vi "ME_acquire_9.vi"() -> ()   [LabVIEW 2015]
doc: "Use this template to build a producer/consumer design pattern. Use this template when you need to execute a process, such as data analysis, when a data source, such as a triggered acquisition, produces data at an uneven rate and you need to execute the process when the data becomes available."
uses:
  Mode.ctl
  oxford_driver/Oxford Drivers/BUSGEN.LLB/OxfordAddress.ctl
  <vilib>/Analysis/baseanly.llb/Mean (DBL).vi
  <vilib>/Utility/file.llb/Write Delimited Spreadsheet (DBL).vi
  <vilib>/express/express arith-compare/Formula/XNode/ExpressFormulaBlockNode.xnode
  <vilib>/Analysis/NI_AALBase.lvlib
panel:
  out "remaining elements":T1(array[cluster])
  in  "Stop":bool
  out "SaveSweep":bool=TRUE
  out "Measurement File_dn":path
  out "Measurement File_up":path
  out "Measurement File_average":path
  out "Actual Polarization":dbl
  in  "Reset IB?":bool
  in  "First?":bool
  in  "Save Period":dbl=1.0
  out "Averaged I(B)":dbl[][](array[numeric])
  out "P(uC/mm^2)":dbl[](array[numeric])
  in  "Sweep Field":bool
  out "P(B)":cluster{"yi":dbl[], dbl[]}(graph)
  out "Offset array":dbl[](array[numeric])
  in  "stop 2":bool
  in  "dB":dbl=0.005
  in  "Dwell Time (ms)":u32=1
  out "appended array":dbl[][](array[numeric])
  in  "Magnet ON?":bool
  out "Actual B Field (T)":dbl
  out "Actual Temperature (K)":dbl
  out "Actual Current (pA)":dbl
  in  "Tab Control":T2(tab)
  out "P(T)":cluster{"yi":dbl[], dbl[]}(graph)
  out "I(T)":cluster{dbl[], dbl[]}(graph)
  in  "Set temperature (K)":dbl=4.5
  in  "Temp Ramping Rate (K/min)":dbl=10.0
  in  "Heater Range":enum16{"Off", "Low", "Medium", "High"}(ring)
  in  "Heater On/Off":bool
  in  "FileName":string
  out "Step Temp":bool
  out "j":i32
  out "i":i32
  in  "Max Countl":i32
  in  "Record ALL":bool
  in  "Sweep Rate Array":dbl[](array[numeric])=[2.0, 1.0, 0.5, 0.1, 0.05, 9.0, 10.0, 11.0, 12.0]
  out "I(B) 3":cluster{dbl[], dbl[]}[](graph)
  in  "Go to Set":bool
  in  "Set Field (T)":dbl
  in  "Field To Zero":bool
  in  "Sweep Rate (T/min)":dbl=2.0 format="%.6f"
  in  "Min Field (T)":dbl
  in  "Max Field (T)":dbl=0.15
  out "Up/Down":bool
  out "I(B) /Averaged/ 2":cluster{"B array":dbl[], dbl[]}[](graph)
  in  "Temperature Array":dbl[](array[numeric])=[4.5, 5.0, 6.0, 7.0, 8.0, 9.0, 10.0, 11.0, 12.0]
  out "New":bool=TRUE
  out "Step Rate":bool
  out "Finished":bool=TRUE
  in  "Directory":string
  out "Wait (s)":dbl
  in  "secs to wait":dbl=180.0
  in  "Measure Noise":bool
  in  "Cycles":i32
  in  "maximum value":dbl=10.0 format="%0.2f"
  in  "minimum value":dbl=-10.0 format="%0.2f"
  in  "physical channels":tag="Dev1/ai1"
  out "PSD (pA/Hz^1/2) Peaks Removed":cluster{"f0":dbl, "df":dbl, "magnitude":dbl[]}(graph)
  out "PSD (pA/Hz^1/2)":cluster{"f0":dbl, "df":dbl, "magnitude":dbl[]}(graph)
  out "Current (pA) Filtered":waveform(dbl)(graph)
  out "Current (pA)":dbl[](graph)
  in  "Samples per channel":i32=1000
  in  "Rate":dbl=1000.0 format="%0.2f"
  in  "Cut-Off Frequency":dbl=100.0 caption="Lower Cut-Off"
  in  "Filter On":bool
  out "Dc offset":dbl
  in  "Calibrate":bool
  in  "IV converter":refnum<visa-resource-name>="GPIB0::20::INSTR"
  in  "Magnetic Field":refnum<visa-resource-name>="GPIB0::21::INSTR"
  out "Time Lag":dbl=0.0500025749206543
  in  "Lake Shore":refnum<visa-resource-name>="GPIB0::11::INSTR"
  in  "Temp Refresh (s)":dbl=0.1
  in  "Sampling rate (Hz)":dbl=10.0
  in  "Gain (V/A)":dbl=1000000000.0
  in  "Sample area (mm^2)":dbl=3.9
  out "B_V":cluster{dbl[], "Best Linear Fit":dbl[]}[](graph)=[{[-0.00854253601, 0.00626134724, 0.0219834428, 0.0379117736, 0.0535871506, 0.0694316728, 0.0851615152, 0.100816481, 0.116478038, 0.132148461, 0.147876163, 0.16341701, 0.178976744, 0.194563632, 0.210251739, 0.225738944, 0.241298253, 0.256806034, 0.272344374, 0.287933477, 0.303494709, 0.318997125, 0.334591297, 0.350146681, 0.365618053, 0.380940961, 0.39666457, 0.412213675, 0.427724671, 0.443221444, 0.458760641, 0.474360042, 0.489915118, 0.505330598, 0.520967119, 0.536347531, 0.551813711, 0.567441155, 0.582995861, 0.598507522, 0.614041988, 0.629563151, 0.645106262, 0.660611914, 0.676136149, 0.691553948, 0.7071244, 0.72262999, 0.738171137, 0.753700392, 0.76919513, 0.784778028, 0.800215944, 0.8156961, 0.831325434, 0.846852183, 0.862326812, 0.877819169, 0.893312568, 0.90888536, 0.924354789], "Best Linear Fit"=[0.0, 0.005, 0.01, 0.015, 0.02, 0.025, 0.03, 0.035, 0.04, 0.045, 0.05, 0.055, 0.06, 0.065, 0.07, 0.075, 0.08, 0.085, 0.09, 0.095, 0.1, 0.105, 0.11, 0.115, 0.12, 0.125, 0.13, 0.135, 0.14, 0.145, 0.15, 0.155, 0.16, 0.165, 0.17, 0.175, 0.18, 0.185, 0.19, 0.195, 0.2, 0.205, 0.21, 0.215, 0.22, 0.225, 0.23, 0.235, 0.24, 0.245, 0.25, 0.255, 0.26, 0.265, 0.27, 0.275, 0.28, 0.285, 0.29, 0.295, 0.3]}, {[-0.00854253601, 0.00626134724, 0.0219834428, 0.0379117736, 0.0535871506, 0.0694316728, 0.0851615152, 0.100816481, 0.116478038, 0.132148461, 0.147876163, 0.16341701, 0.178976744, 0.194563632, 0.210251739, 0.225738944, 0.241298253, 0.256806034, 0.272344374, 0.287933477, 0.303494709, 0.318997125, 0.334591297, 0.350146681, 0.365618053, 0.380940961, 0.39666457, 0.412213675, 0.427724671, 0.443221444, 0.458760641, 0.474360042, 0.489915118, 0.505330598, 0.520967119, 0.536347531, 0.551813711, 0.567441155, 0.582995861, 0.598507522, 0.614041988, 0.629563151, 0.645106262, 0.660611914, 0.676136149, 0.691553948, 0.7071244, 0.72262999, 0.738171137, 0.753700392, 0.76919513, 0.784778028, 0.800215944, 0.8156961, 0.831325434, 0.846852183, 0.862326812, 0.877819169, 0.893312568, 0.90888536, 0.924354789], "Best Linear Fit"=[-0.00022554388023060128, 0.004536267537808887, 0.009593430775915074, 0.014716931562355689, 0.01975906732634002, 0.024855610270593523, 0.029915265354287977, 0.03495083565949541, 0.03998852608757118, 0.045029068349812316, 0.05008803495326229, 0.055086897848955874, 0.060091835929837946, 0.06510550835596321, 0.07015173884687344, 0.07513334727738563, 0.08013814865293042, 0.08512637555172443, 0.0901244320467579, 0.09513881694893507, 0.10014423687592358, 0.10513073807087174, 0.11014675346564809, 0.1151502923271957, 0.12012680792099008, 0.1250555686413888, 0.1301132186920259, 0.13511473785283767, 0.14010399888730068, 0.14508868495702945, 0.1500870171143548, 0.15510471446726903, 0.16010815425765457, 0.16506669165212906, 0.17009632901003072, 0.1750435864450521, 0.18001843198211442, 0.1850451496356715, 0.19004847041199868, 0.1950379453501071, 0.20003475573578386, 0.20502728708357412, 0.21002687821664084, 0.21501442030211, 0.220007939788244, 0.2249672231113706, 0.22997560874002893, 0.23496313088260184, 0.23996209027618054, 0.24495722449359253, 0.24994125598600042, 0.2549536449902534, 0.25991939913989753, 0.2648987401917687, 0.26992606578200207, 0.2749203939204135, 0.2798979571595809, 0.2848812227804405, 0.2898648235706211, 0.2948739618827834, 0.2998498524919418]}]
  out "V_I":cluster{dbl[], "Best Linear Fit":dbl[]}[](graph)=[{[0.0, 0.035, 0.069, 0.104, 0.138, 0.173, 0.208, 0.242, 0.277, 0.311, 0.346, 0.38, 0.415, 0.45, 0.484, 0.519, 0.553, 0.588, 0.623, 0.657, 0.692, 0.726, 0.761, 0.796, 0.83, 0.865, 0.899, 0.934, 0.969, 1.003, 1.038, 1.072, 1.107, 1.141, 1.176, 1.211, 1.245, 1.28, 1.314, 1.349, 1.384, 1.418, 1.453, 1.487, 1.522, 1.557, 1.591, 1.626, 1.66, 1.695, 1.73, 1.764, 1.799, 1.833, 1.868, 1.902, 1.937, 1.972, 2.006, 2.041, 2.075], "Best Linear Fit"=[-0.00854253601, 0.00626134724, 0.0219834428, 0.0379117736, 0.0535871506, 0.0694316728, 0.0851615152, 0.100816481, 0.116478038, 0.132148461, 0.147876163, 0.16341701, 0.178976744, 0.194563632, 0.210251739, 0.225738944, 0.241298253, 0.256806034, 0.272344374, 0.287933477, 0.303494709, 0.318997125, 0.334591297, 0.350146681, 0.365618053, 0.380940961, 0.39666457, 0.412213675, 0.427724671, 0.443221444, 0.458760641, 0.474360042, 0.489915118, 0.505330598, 0.520967119, 0.536347531, 0.551813711, 0.567441155, 0.582995861, 0.598507522, 0.614041988, 0.629563151, 0.645106262, 0.660611914, 0.676136149, 0.691553948, 0.7071244, 0.72262999, 0.738171137, 0.753700392, 0.76919513, 0.784778028, 0.800215944, 0.8156961, 0.831325434, 0.846852183, 0.862326812, 0.877819169, 0.893312568, 0.90888536, 0.924354789]}, {[0.0, 0.035, 0.069, 0.104, 0.138, 0.173, 0.208, 0.242, 0.277, 0.311, 0.346, 0.38, 0.415, 0.45, 0.484, 0.519, 0.553, 0.588, 0.623, 0.657, 0.692, 0.726, 0.761, 0.796, 0.83, 0.865, 0.899, 0.934, 0.969, 1.003, 1.038, 1.072, 1.107, 1.141, 1.176, 1.211, 1.245, 1.28, 1.314, 1.349, 1.384, 1.418, 1.453, 1.487, 1.522, 1.557, 1.591, 1.626, 1.66, 1.695, 1.73, 1.764, 1.799, 1.833, 1.868, 1.902, 1.937, 1.972, 2.006, 2.041, 2.075], "Best Linear Fit"=[-0.007846580254753975, 0.007882153481927697, 0.02316149482613275, 0.03889022856281441, 0.054169569907019474, 0.06989830364370113, 0.08562703738038281, 0.10090637872458785, 0.11663511246126955, 0.1319144538054746, 0.14764318754215625, 0.1629225288863613, 0.17865126262304296, 0.19437999635972467, 0.2096593377039297, 0.22538807144061138, 0.24066741278481643, 0.25639614652149806, 0.27212488025817977, 0.2874042216023848, 0.3031329553390665, 0.31841229668327153, 0.3341410304199532, 0.3498697641566349, 0.3651491055008399, 0.3808778392375216, 0.39615718058172666, 0.4118859143184083, 0.42761464805509, 0.442893989399295, 0.45862272313597674, 0.4739020644801818, 0.48963079821686345, 0.5049101395610684, 0.5206388732977502, 0.5363676070344319, 0.5516469483786369, 0.5673756821153185, 0.5826550234595236, 0.5983837571962053, 0.6141124909328869, 0.629391832277092, 0.6451205660137737, 0.6603999073579787, 0.6761286410946604, 0.691857374831342, 0.7071367161755471, 0.7228654499122288, 0.7381447912564338, 0.7538735249931156, 0.7696022587297972, 0.7848816000740022, 0.8006103338106839, 0.815889675154889, 0.8316184088915707, 0.8468977502357756, 0.8626264839724573, 0.878355217709139, 0.893634559053344, 0.9093632927900257, 0.9246426341342309]}]
  out "B0 (T)":dbl=0.0025222449819540214
  out "B/V (T/V)":dbl=0.321659617116981
  out "I0 (A)":dbl=-0.007846580254753975
  out "V/I (Ohm)":dbl=0.44939239247661916
  in  "Offset?":bool
  in  "Temp/Magnetic Field":bool
  out "index":i8
  out "Read?":bool
  out "Magnetic Field (T)":dbl[](array[numeric])
  out "Reset":bool
  out "Measured Current (pA)":dbl[](array[numeric])
  out "Elapsed Time (s)":dbl[](array[numeric])
  out "Start time":timestamp
  in  "Enum":T3=enum."Process"
  out "B array":dbl[](array[numeric])
  in  "dB (T)":dbl=0.0025
  in  "Counter":i8
  out "L magnet (H)":dbl
  out "R magnet (mOhm)":dbl
  out "Actual Current (R0)":dbl
  out "Actual Field (T)":dbl
  out "Temperature array":dbl[](array[numeric])
  in  "New Measurement File":bool
  out "Measurement File":path
  out "refnum out":refnum<file>
  in  "Measuring":bool
  in  "Measure /Pause":bool
  in  "stop":bool
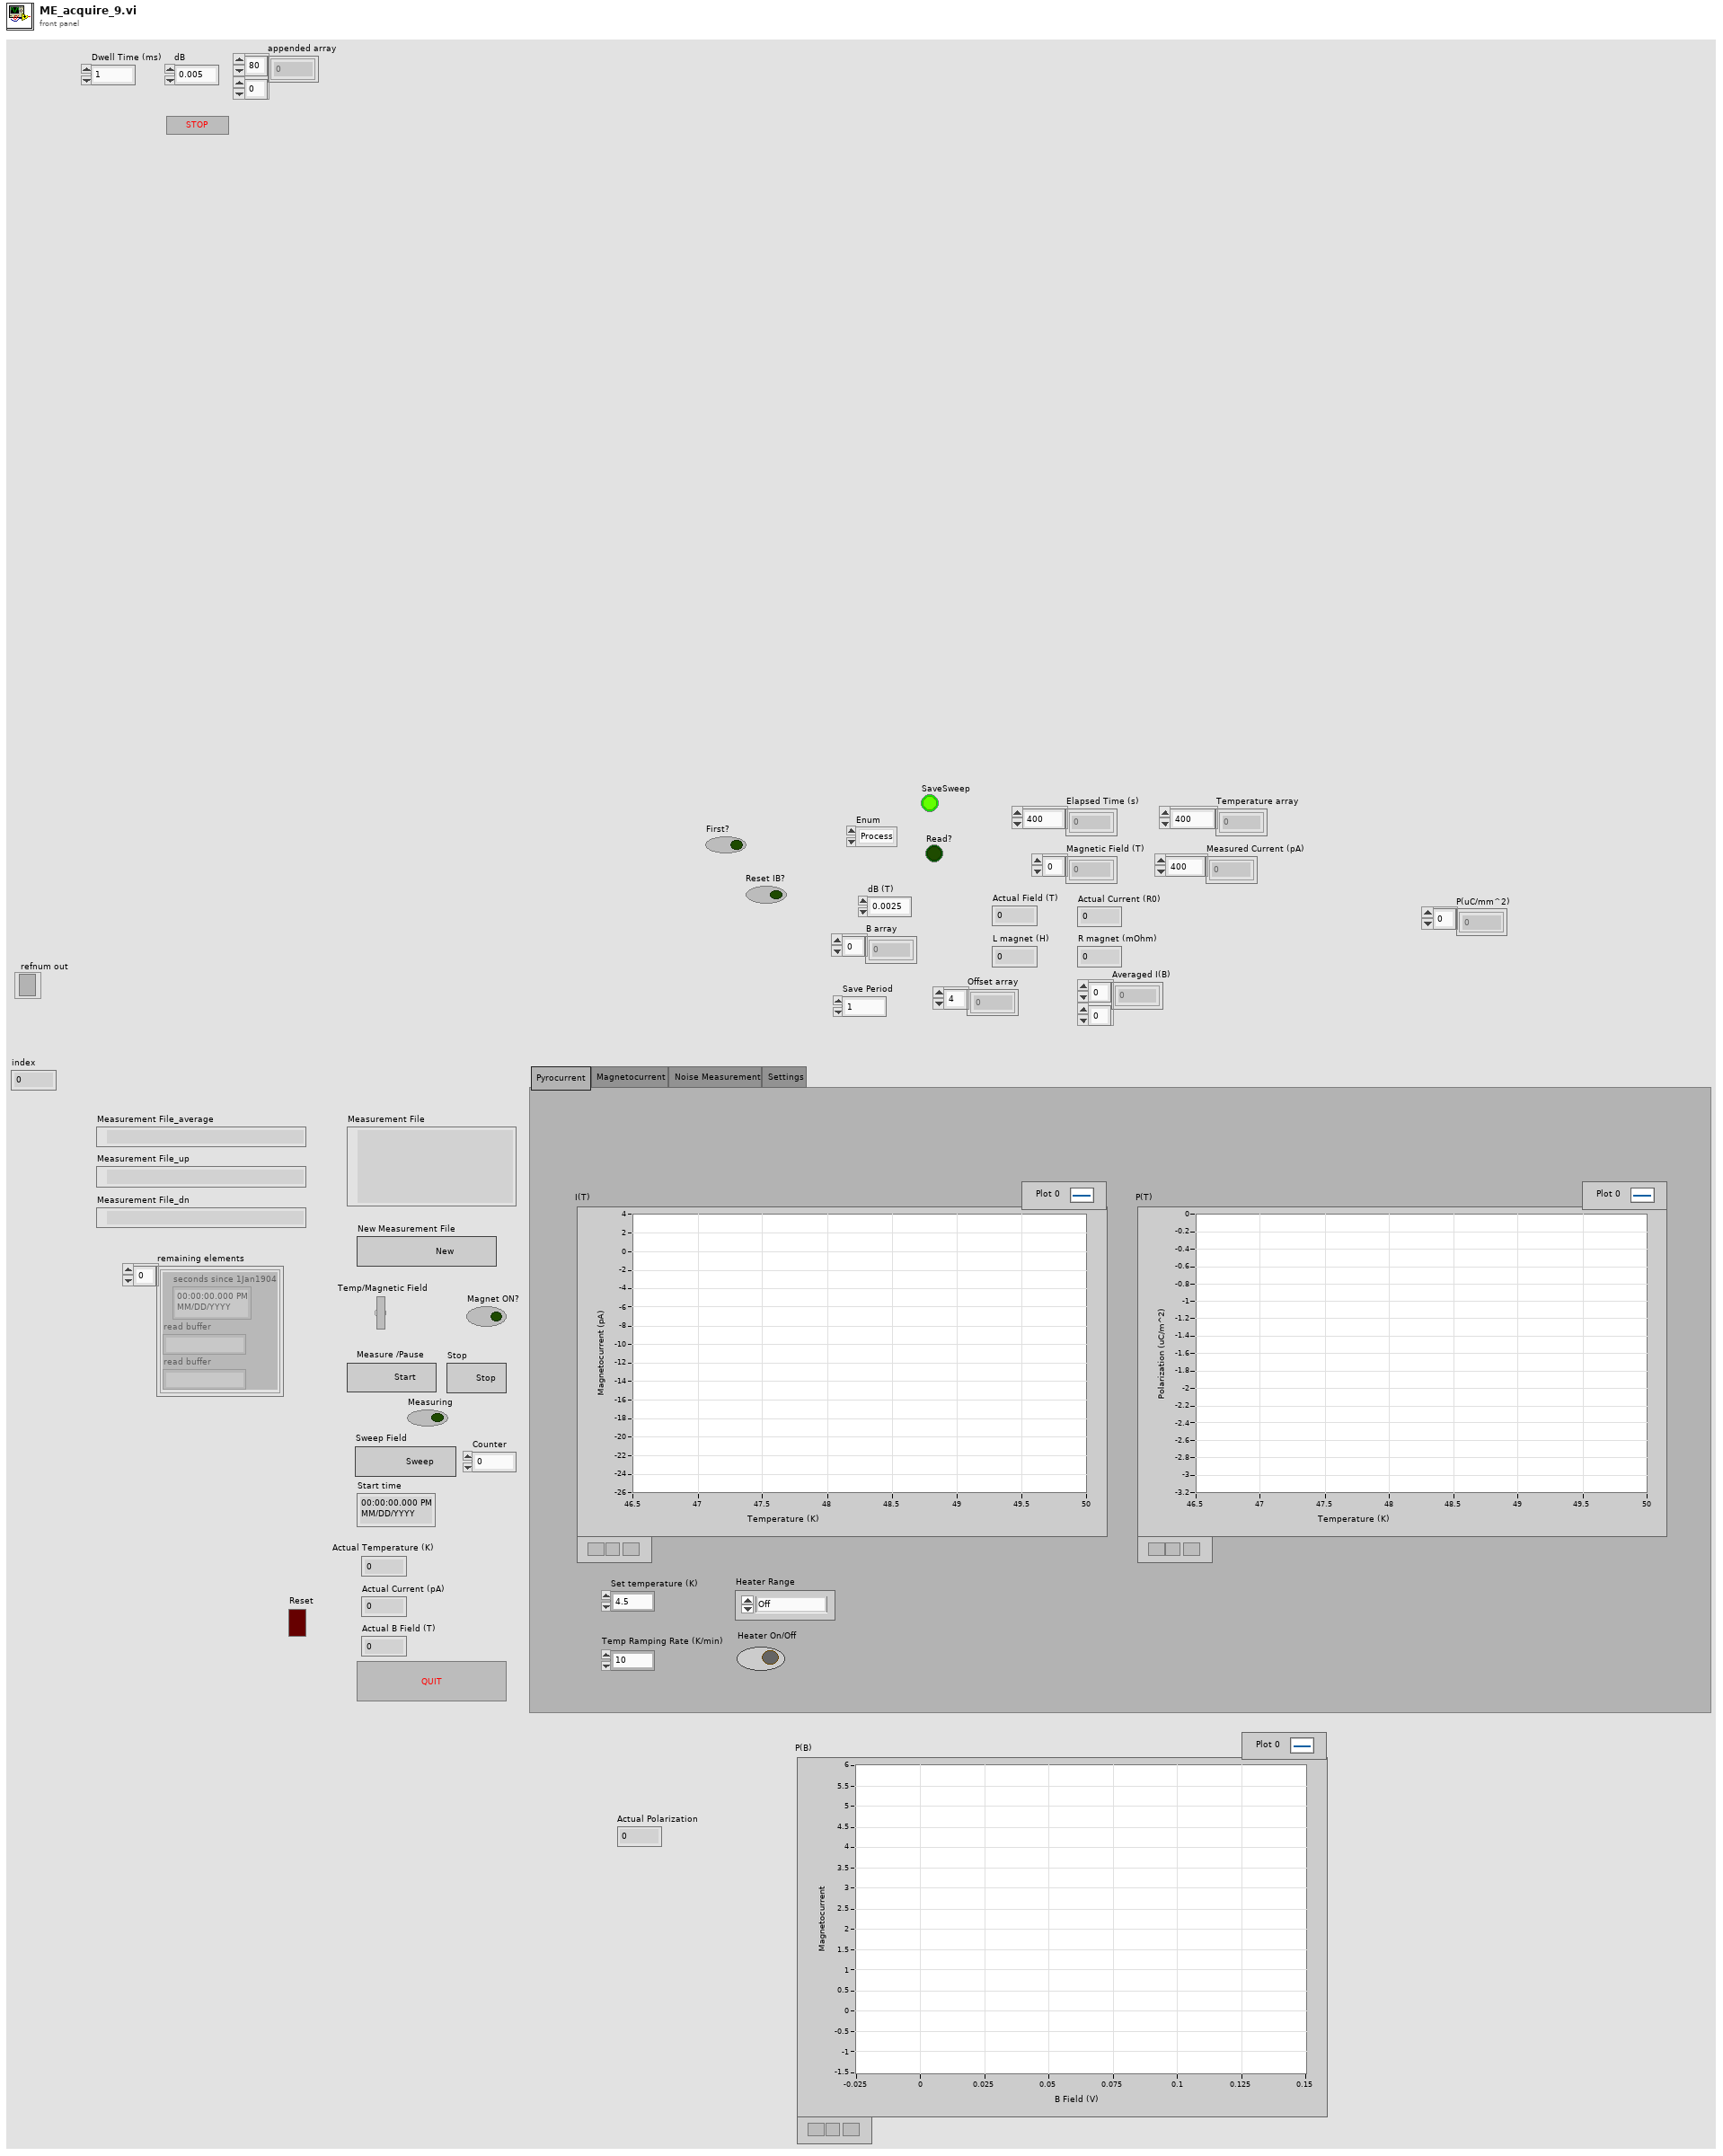
[diagram p1: front panel]
types:
  T1 = cluster{"seconds since 1Jan1904":timestamp, "read buffer":string, "read buffer":string}[]
  T2 = enum32{"Pyrocurrent", "Magnetocurrent", "Noise Measurement", "Settings"}
  T3 = typedef "Mode.ctl" = enum16{"Offset", "Process", "Sweep", "Plot", "Save", "New", "Return", ""}
  T4 = enum16{"open", "replace", "create", "open or create", "replace or create", "replace or create with confirmation"}
  T5 = typedef "OxfordAddress.ctl" = cluster{"Com Port":i32, "ISOBUS Address":i32, "GPIB Address":i16, "Communication":enum16{"RS232", "ISOBUS", "GPIB", "Gateway"}}
  T6 = cluster{"seconds since 1Jan1904":timestamp, "read buffer":string, "read buffer":string}
  T7 = cluster{"B array":dbl[], "Averaged I(B) out":dbl[]}
  T8 = cluster{"B array":dbl[], "Averaged I(B) out":dbl[]}[]
  T9 = cluster{"I array out (A)":dbl[], "V array out (V)":dbl[]}
  T10 = cluster{"I array out (A)":dbl[], "Best Linear Fit":dbl[]}
  T11 = cluster{"V array out (V)":dbl[], "B array Out":dbl[]}
  T12 = cluster{"V array out (V)":dbl[], "Best Linear Fit 2":dbl[]}
  T13 = cluster{"I array out (A)":dbl[], "Best Linear Fit":dbl[]}[]
  T14 = cluster{"V array out (V)":dbl[], "Best Linear Fit 2":dbl[]}[]
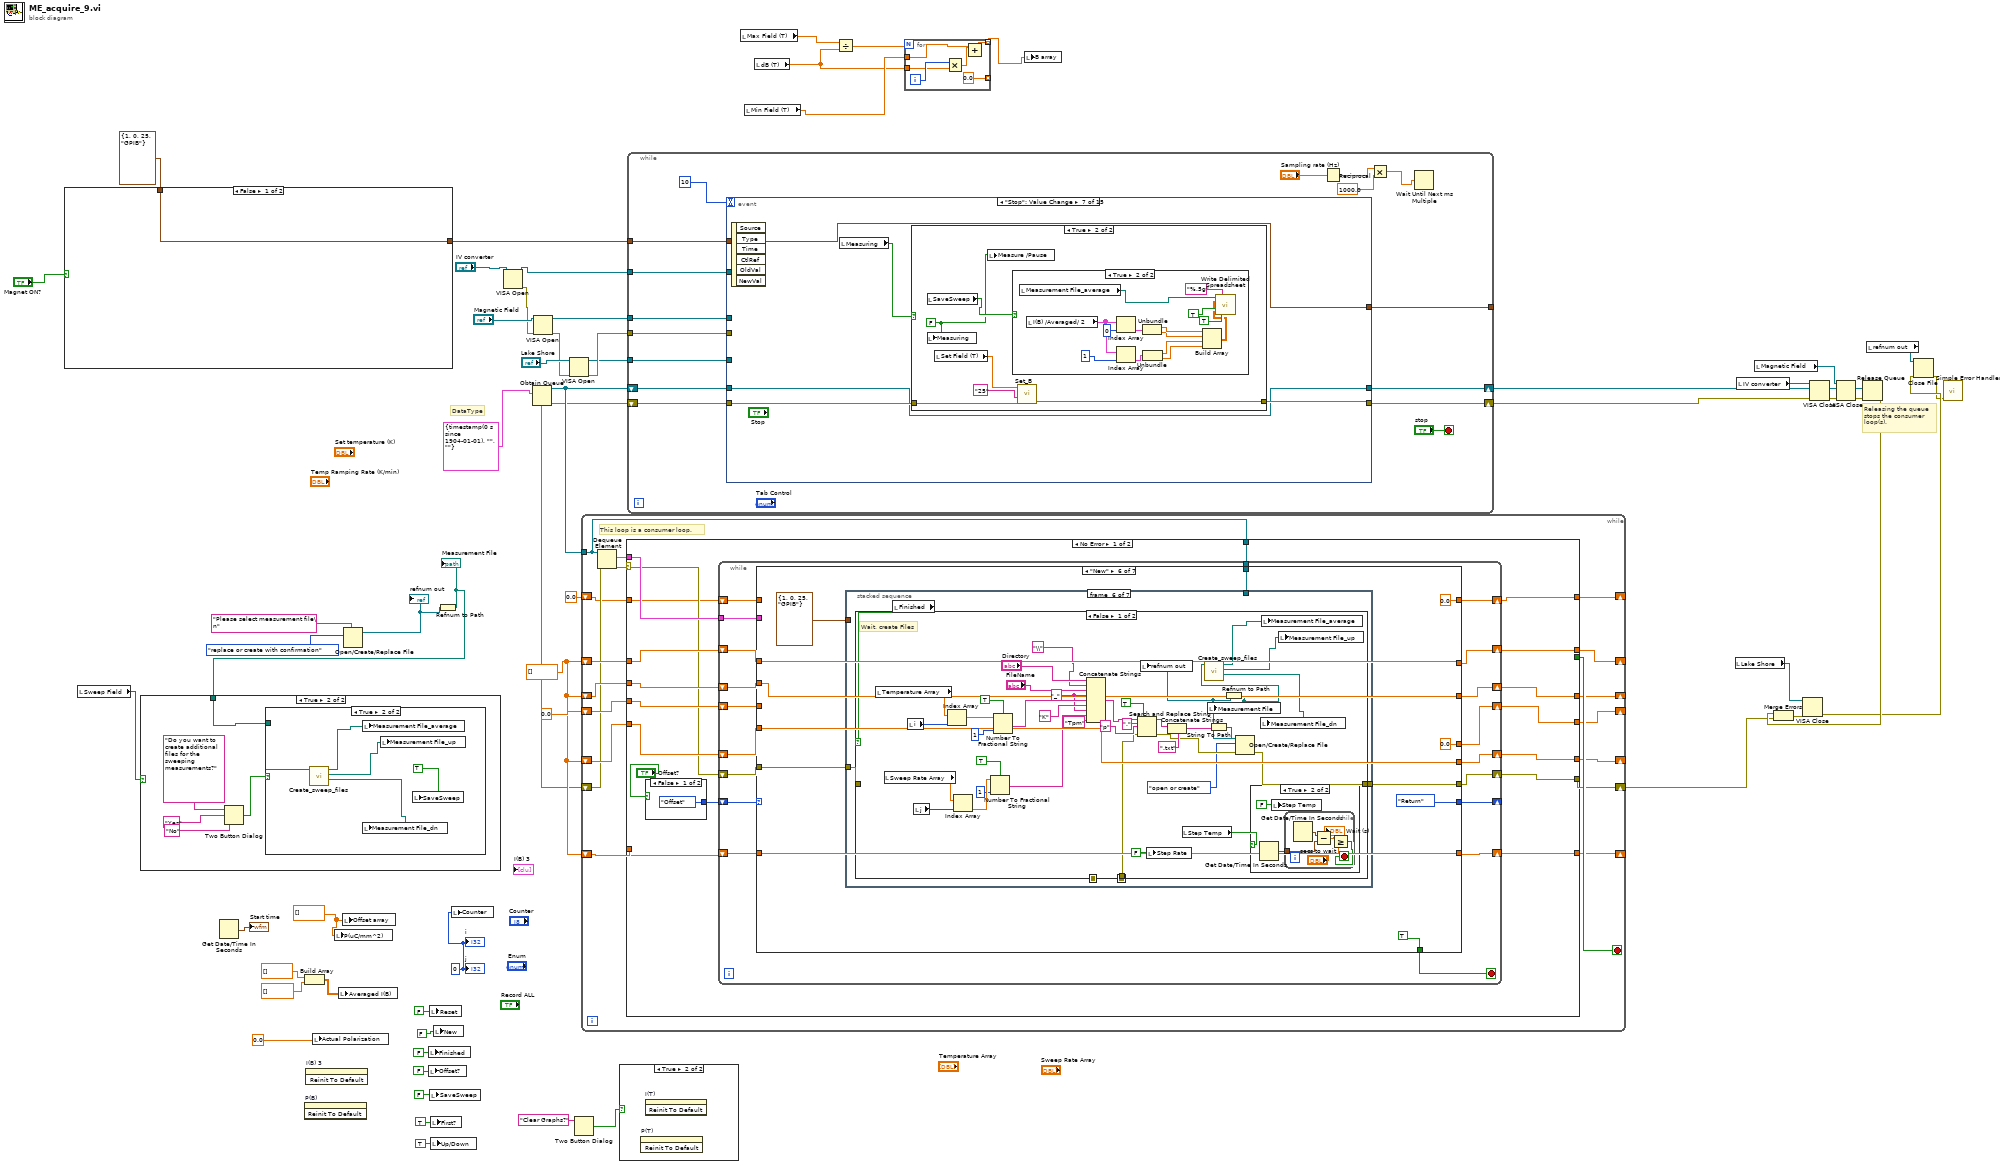
[diagram p0: block diagram]
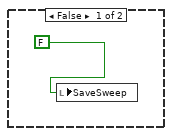
[diagram p4: hidden frame]
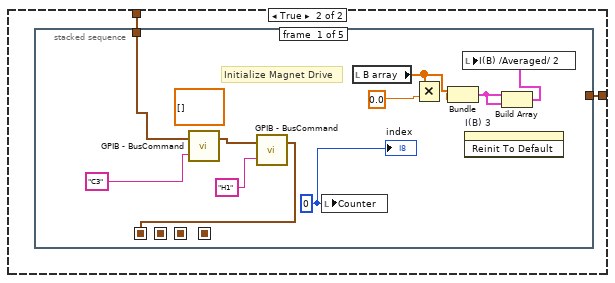
[diagram p5: hidden frame]
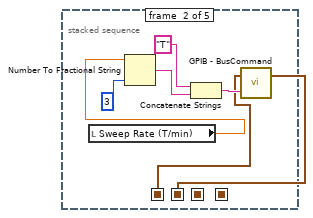
[diagram p6: hidden frame]
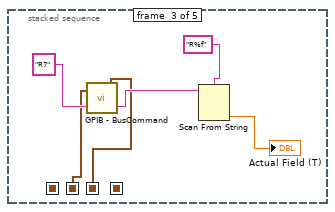
[diagram p7: hidden frame]
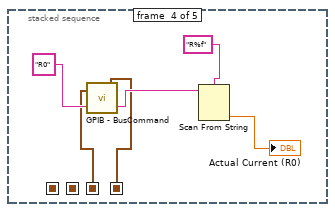
[diagram p8: hidden frame]
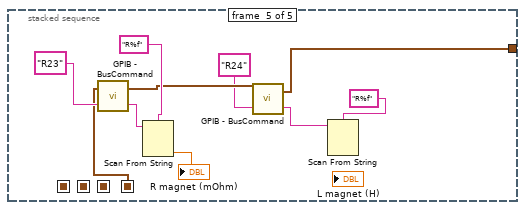
[diagram p9: hidden frame]
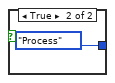
[diagram p10: hidden frame]
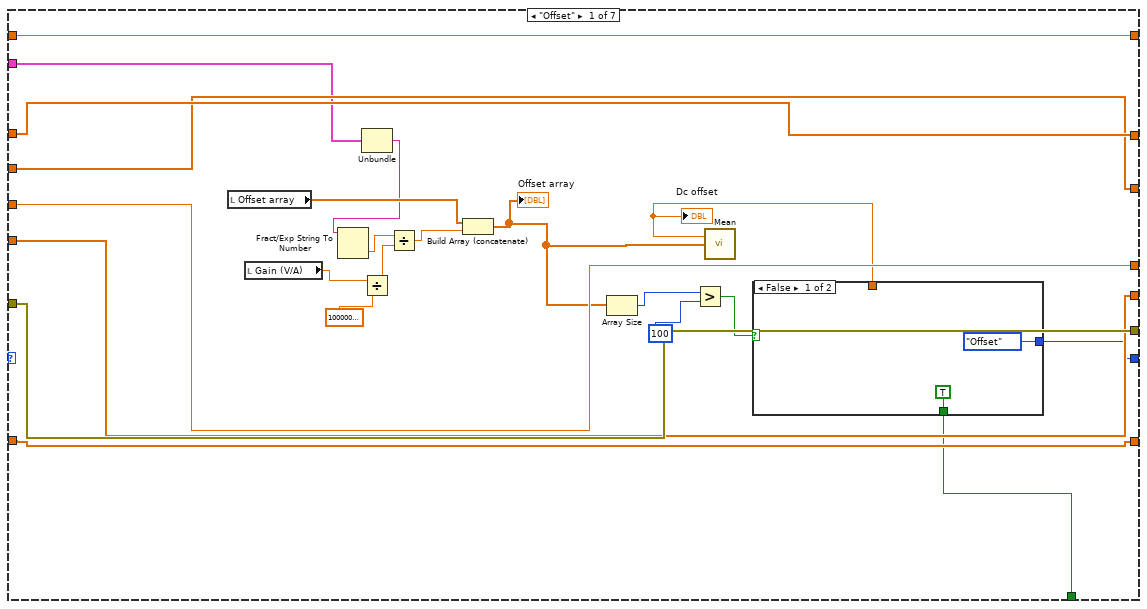
[diagram p11: hidden frame]
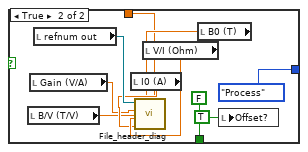
[diagram p12: hidden frame]
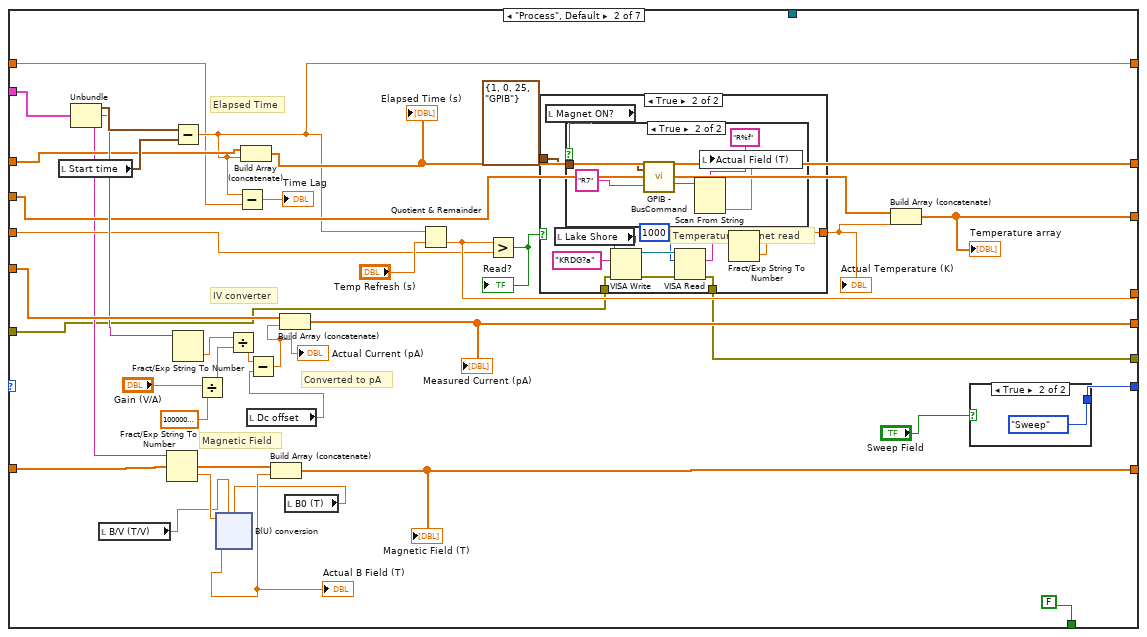
[diagram p13: hidden frame]
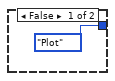
[diagram p14: hidden frame]
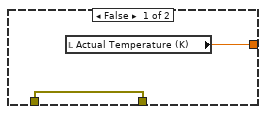
[diagram p15: hidden frame]
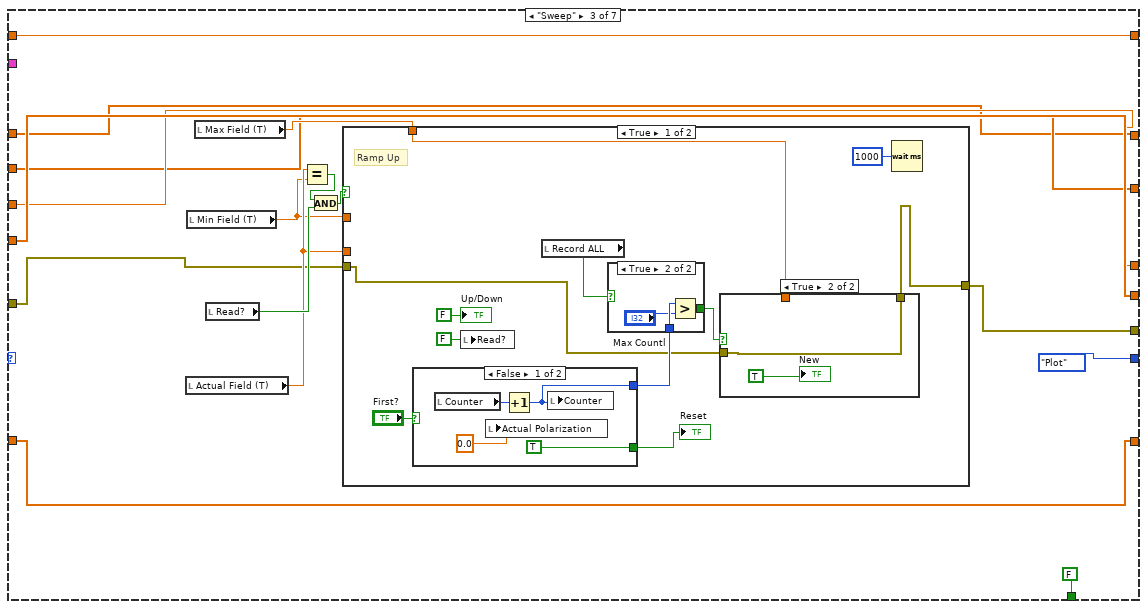
[diagram p17: hidden frame]
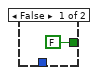
[diagram p18: hidden frame]
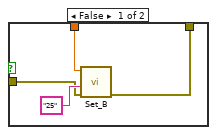
[diagram p19: hidden frame]
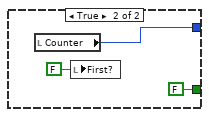
[diagram p20: hidden frame]
diagram:
  w3 = 0 ("j")
  w22 = dbl[] []
  w28 = dbl[] []
  # "DataType"
  # "Releasing the queue stops the consumer loop(s)."
  n1 = case shown="False" "Magnet ON?" {
    tunnel: T5 {"Com Port"=1, "ISOBUS Address"=0, "GPIB Address"=25, "Communication"=enum."GPIB"} ("Address") -> [w58 w60]
    tunnel: [w58 w59] -> w36
    frame False {
    }
    frame True {
      n2 = stacked-sequence {
        seq-local: [w68 _ _ _ _] -> [_ w73 _ _ _]
        seq-local: [_ w72 _ _ _] -> [_ _ w80 _ _]
        seq-local: [_ _ w79 _ _] -> [_ _ _ w86 _]
        seq-local: [_ _ _ w85 _] -> [_ _ _ _ w96]
        tunnel: w60 -> [w70 _ _ _ _]
        tunnel: [_ _ _ _ w94] -> w59
        frame #0 {
          (unwired) dbl[][] []
          w66 = i8 0 ("Counter")
          # "Initialize Magnet Drive"
          n3 = call "GPIB - BusCommand.vi"("Command"="C3", "Address"=w70) -> ("Address(thru)"=w69:T5)  [unwired: 1 out]
          n4 = call "GPIB - BusCommand.vi"("Command"="H1", "Address"=w69) -> ("Address(thru)"=w68:T5)  [unwired: 1 out]
          n5 = local write "Counter"(w66) -> ()
          n6 = local read "B array"() -> (w64:dbl[])
          n7 = Multiply(x=w64, y=0.0) -> (x*y=w63:dbl[])
          n8 = Bundle("B array"=w64, w63) -> (w62:cluster{"B array":dbl[], dbl[]})  [unwired: 1 in]
          n9 = invoke on="I(B) 3" class="XYGraph (strict)" method="Reinit To Default"() -> ()  [unwired: 3 in, 3 out]
          n10 = Build Array(w62, w62) -> (w61:cluster{"B array":dbl[], dbl[]}[])
          n11 = local write "I(B) /Averaged/ 2"(w61) -> ()
          "index" <- w66
        }
        frame #1 {
          n12 = local read "Sweep Rate (T/min)"() -> (w74:dbl)
          n13 = Number To Fractional String(number=w74, precision (6)=i16 3) -> (F-format string=w76:string)  [unwired: 2 in]
          n14 = Concatenate Strings("T" ("format string"), w76) -> (w75:string)
          n15 = call "GPIB - BusCommand.vi"("Command"=w75, "Address"=w73) -> ("Address(thru)"=w72:T5)  [unwired: 1 out]
        }
        frame #2 {
          n16 = call "GPIB - BusCommand.vi"("Command"="R7" ("format string"), "Address"=w80) -> ("Reply"=w84:string, "Address(thru)"=w79:T5)
          n17 = Scan From String(format string="R%f" ("remaining string"), input string=w84) -> (output 1=→"Actual Field (T)":dbl)  [unwired: 3 in, 3 out]
        }
        frame #3 {
          n18 = call "GPIB - BusCommand.vi"("Command"="R0" ("format string"), "Address"=w86) -> ("Reply"=w90:string, "Address(thru)"=w85:T5)
          n19 = Scan From String(format string="R%f" ("remaining string"), input string=w90) -> (output 1=→"Actual Current (R0)":dbl)  [unwired: 3 in, 3 out]
        }
        frame #4 {
          n20 = call "GPIB - BusCommand.vi"("Command"="R23" ("format string"), "Address"=w96) -> ("Reply"=w100:string, "Address(thru)"=w95:T5)
          n21 = Scan From String(format string="R%f" ("remaining string"), input string=w100) -> (output 1=→"R magnet (mOhm)":dbl)  [unwired: 3 in, 3 out]
          n22 = call "GPIB - BusCommand.vi"("Command"="R24" ("format string"), "Address"=w95) -> ("Reply"=w92:string, "Address(thru)"=w94:T5)
          n23 = Scan From String(format string="R%f" ("remaining string"), input string=w92) -> ()  [unwired: 4 in, 3 out]
        }
      }
    }
  }
  n24 = local read "Sweep Field"() -> (w8:bool)
  n25 = Get Date/Time In Seconds() -> (seconds since 1Jan1904=→"Start time":timestamp)
  n26 = Build Array(dbl[] [], dbl[] []) -> (w19:dbl[][])
  n27 = invoke on="P(B)" class="XYGraph (strict)" method="Reinit To Default"() -> ()  [unwired: 3 in, 3 out]
  n28 = invoke on="I(B) 3" class="XYGraph (strict)" method="Reinit To Default"() -> ()  [unwired: 3 in, 3 out]
  n29 = local write "Actual Polarization"(0.0 ("Actual Polarization")) -> ()
  n30 = local write "P(uC/mm^2)"(w22) -> ()
  n31 = local write "Averaged I(B)"(w19) -> ()
  n32 = local write "Offset array"(w22) -> ()
  n33 = Open/Create/Replace File(prompt="Please select measurement file\n", operation (0:open)=T4."replace or create with confirmation") -> (refnum out=w33:refnum<file>)  [unwired: 4 in, 2 out]
  "refnum out" <- w33
  n34 = local write "Finished"(FALSE ("Finished")) -> ()
  n35 = local write "Offset?"(FALSE ("Offset?")) -> ()
  n36 = local write "Reset"(FALSE ("Reset")) -> ()
  n37 = local write "SaveSweep"(FALSE ("SaveSweep")) -> ()
  n38 = local write "First?"(TRUE ("First?")) -> ()
  n39 = local write "Up/Down"(TRUE ("Up/Down")) -> ()
  n40 = local write "New"(FALSE ("New")) -> ()
  n41 = Refnum to Path(1:w33) -> (0:w7:path)
  "Measurement File" <- w7
  n42 = case shown="True" w8 {
    tunnel: w7 -> [_ w101]
    frame False {
    }
    frame True {
      n43 = Two Button Dialog(message="Do you want to create additional files for the sweeping measurements?" ("string"), 1:"No" ("F button name (\"Cancel\")"), 2:"Yes" ("T button name (\"OK\")")) -> (T button?=w103:bool)
      n44 = case shown="True" w103 {
        tunnel: w101 -> [_ w111]
        frame False {
          n45 = local write "SaveSweep"(FALSE ("SaveSweep")) -> ()
        }
        frame True {
          n46 = call "Create_sweep_files.vi"("Measurement File"=w111) -> ("Path 3"=w108:path, "Path 2"=w109:path, "Path"=w110:path)  [unwired: 8 in]
          n47 = local write "Measurement File_dn"(w108) -> ()
          n48 = local write "Measurement File_average"(w110) -> ()
          n49 = local write "Measurement File_up"(w109) -> ()
          n50 = local write "SaveSweep"(TRUE) -> ()
        }
      }
    }
  }
  n51 = local write "Counter"(w3) -> ()
  n52 = VISA Open(VISA resource name="IV converter") -> (VISA resource name=w52:refnum<visa-resource-name>, error out=w54:errorcluster)  [unwired: 4 in]
  n53 = Obtain Queue(element data type=T6 {"seconds since 1Jan1904"=timestamp(0 s since 1904-01-01), "read buffer"="", "read buffer"=""} ("output cluster")) -> (queue out=w57:refnum<queue>, error out=w26:errorcluster)  [unwired: 4 in, 1 out]
  n54 = VISA Open(error in (no error)=w54, VISA resource name="Magnetic Field") -> (VISA resource name=w51:refnum<visa-resource-name>, error out=w30:errorcluster)  [unwired: 3 in]
  n55 = VISA Open(error in (no error)=w30, VISA resource name="Lake Shore") -> (VISA resource name=w24:refnum<visa-resource-name>, error out=w29:errorcluster)  [unwired: 3 in]
  n56 = Two Button Dialog(message="Clear Graphs?") -> (T button?=w2:bool)  [unwired: 2 in]
  n57 = while {
    tunnel: w57 -> [w112]
    shift-right: [w125] -> _
    shift-left: w28 -> [w124]
    shift-right: [w123] -> _
    shift-left: w28 -> [w122]
    shift-right: [w121] -> _
    shift-left: w28 -> [w120]
    shift-right: [w119] -> _
    shift-left: 0.0 -> [w118]
    shift-right: [w117] -> _
    shift-left: w28 -> [w116]
    shift-right: [w126] -> w41
    shift-left: w26 -> [w115]
    shift-right: [w114] -> _
    shift-left: 0.0 -> [w113]
    stop <- w127 stop-if-true
    # "This loop is a consumer loop."
    n58 = Dequeue Element(queue=w112, error in (no error)=w115) -> (element=w128:T6, error out=w129:errorcluster)  [unwired: 1 in, 2 out]
    n59 = case shown="No Error" w129 {
      selector: w129 -> [w135 w640]
      tunnel: w128 -> [w146 _]
      tunnel: [_ TRUE] -> w127
      tunnel: [w134 w640] -> w126
      tunnel: [w145 w639] -> w125
      tunnel: w124 -> [w144 w639]
      tunnel: [w143 w636] -> w123
      tunnel: w122 -> [w142 w636]
      tunnel: [w141 w635] -> w121
      tunnel: w120 -> [w140 w635]
      tunnel: [w139 w637] -> w119
      tunnel: w118 -> [w138 w637]
      tunnel: [w137 w638] -> w117
      tunnel: w116 -> [w136 w638]
      tunnel: [w133 w634] -> w114
      tunnel: w113 -> [w132 w634]
      tunnel: w112 -> [w130 _]
      frame No Error {
        n60 = case shown="False" "Offset?" {
          tunnel: [Mode."Offset" ("Enum") Mode."Process" ("Enum")] -> w147
          frame False {
          }
          frame True {
          }
        }
        n61 = while {
          shift-right: [w156] -> _
          shift-left: w147 -> [w168]
          tunnel: w146 -> [w167]
          shift-right: [w166] -> w145
          shift-left: w144 -> [w165]
          shift-right: [w158] -> w137
          shift-left: w136 -> [w157]
          shift-right: [w160] -> w139
          shift-left: w138 -> [w159]
          shift-right: [w164] -> w143
          shift-left: w142 -> [w163]
          shift-right: [w154] -> w134
          shift-left: w135 -> [w155]
          shift-right: [w162] -> w141
          shift-left: w140 -> [w161]
          shift-right: [w152] -> w133
          shift-left: w132 -> [w151]
          tunnel: w130 -> [w150]
          stop <- w153 stop-if-true
          n62 = case shown="\"New\"" w168 {
            selector: w168 -> [_ _ _ _ _ _ w627]
            tunnel: w167 -> [w184 w238 _ _ _ _ _]
            tunnel: [w190 w235 w275 w343 w416 w484 w632] -> w166
            tunnel: w165 -> [w190 w226 w275 w343 w412 w484 w632]
            tunnel: [w185 w234 w278 w345 w418 w482 w629] -> w164
            tunnel: w163 -> [w185 w233 w278 w345 w413 w482 w629]
            tunnel: [w186 w230 w280 w340 w419 w480 w626] -> w162
            tunnel: w161 -> [w186 w229 w280 w340 w414 w480 w626]
            tunnel: [w188 w225 w277 w341 w422 0.0 w630] -> w160
            tunnel: w159 -> [w188 w224 w277 w341 w422 _ w630]
            tunnel: [w189 w221 w276 w342 w417 w483 w631] -> w158
            tunnel: w157 -> [w189 w222 w276 w342 w415 w483 w631]
            tunnel: [w173 w219 Mode."Plot" ("Enum") Mode."Save" ("Enum") w423 Mode."Return" ("Enum") w627] -> w156
            tunnel: w155 -> [w187 w217 w282 w348 w421 w476 w628]
            tunnel: [w187 w216 w281 w348 w421 w475 w628] -> w154
            tunnel: [w169 FALSE FALSE FALSE w410 TRUE TRUE] -> w153
            tunnel: [w172 w213 w274 w344 w420 0.0 w633] -> w152
            tunnel: w151 -> [w172 w212 w274 w344 w420 _ w633]
            tunnel: w150 -> [_ _ _ _ _ w474 _]
            frame "Offset" {
              n63 = local read "Offset array"() -> (w178:dbl[])
              n64 = local read "Gain (V/A)"() -> (w182:dbl)
              n65 = Unbundle(w184) -> ("read buffer"=w171:string)  [unwired: 2 out]
              n66 = Fract/Exp String To Number(string=w171) -> (number=w183:dbl)  [unwired: 3 in, 1 out]
              n67 = Divide(x=w182, y=1000000000000.0) -> (x/y=w180:dbl)
              n68 = Divide(x=w183, y=w180) -> (x/y=w179:dbl)
              n69 = Build Array (concatenate)(w178, w179) -> (w174:dbl[])
              "Offset array" <- w174
              n70 = Array Size(array=w174) -> (size(s)=w177:i32)
              n71 = Greater?(x=w177, y=100) -> (0:w175:bool)
              n72 = call-poly <vilib>:"Mean.vi"("X"=w174) -> ("mean"=w170:dbl)  [unwired: 1 out]
              "Dc offset" <- w170
              n73 = case shown="False" w175 {
                tunnel: [Mode."Offset" ("Enum") Mode."Process" ("Enum")] -> w173
                tunnel: w170 -> [_ w194]
                tunnel: [TRUE FALSE] -> w169
                frame False {
                }
                frame True {
                  n74 = local read "B/V (T/V)"() -> (w195:dbl)
                  n75 = local read "Gain (V/A)"() -> (w196:dbl)
                  n76 = local read "refnum out"() -> (w200:refnum<file>)
                  n77 = local read "I0 (A)"() -> (w198:dbl)
                  n78 = local read "V/I (Ohm)"() -> (w199:dbl)
                  n79 = local read "B0 (T)"() -> (w197:dbl)
                  n80 = call "File_header_diag.vi"("OFFSET"=w194, "B0"=w197, "B/V"=w195, "I0"=w198, "V/I"=w199, "Gain"=w196, "Byte Stream File in"=w200) -> ()  [unwired: 5 in]
                  n81 = local write "Offset?"(TRUE ("Offset?")) -> ()
                }
              }
            }
            frame "Process", Default {
              # "Converted to pA"
              # "Magnetic Field"
              # "IV converter"
              # "Elapsed Time"
              n82 = local read "Start time"() -> (w236:timestamp)
              n83 = Unbundle(w238) -> ("seconds since 1Jan1904"=w237:timestamp, "read buffer"=w231:string, "read buffer"=w218:string)
              n84 = local read "B/V (T/V)"() -> (w208:dbl)
              n85 = Fract/Exp String To Number(string=w218) -> (number=w228:dbl)  [unwired: 3 in, 1 out]
              n86 = Subtract(x=w237, y=w236) -> (x-y=w213:dbl)
              n87 = Fract/Exp String To Number(string=w231) -> (number=w232:dbl)  [unwired: 3 in, 1 out]
              n88 = Divide(x="Gain (V/A)", y=1000000000000.0) -> (x/y=w211:dbl)
              n89 = Divide(x=w232, y=w211) -> (x/y=w206:dbl)
              n90 = Subtract(x=w213, y=w212) -> (x-y=→"Time Lag":dbl)
              n91 = Build Array (concatenate)(w226, w213) -> (w235:dbl[])
              "Elapsed Time (s)" <- w235
              n92 = local read "Dc offset"() -> (w204:dbl)
              n93 = Subtract(x=w206, y=w204) -> (x-y=w205:dbl)
              "Actual Current (pA)" <- w205
              n94 = Build Array (concatenate)(w233, w205) -> (w234:dbl[])
              "Measured Current (pA)" <- w234
              n95 = local read "B0 (T)"() -> (w207:dbl)
              n96 = xnode "B(U) conversion"("V"=w228, "BpV"=w208, "B0"=w207) -> ("Result"=w227:dbl)  [unwired: 1 in, 1 out]
              "Actual B Field (T)" <- w227
              n97 = Build Array (concatenate)(w229, w227) -> (w230:dbl[])
              "Magnetic Field (T)" <- w230
              n98 = Quotient & Remainder(x=w213, y="Temp Refresh (s)") -> (floor(x/y)=w225:dbl)  [unwired: 1 out]
              n99 = Greater?(x=w225, y=w224) -> (0:w223:bool)
              "Read?" <- w223
              n100 = case shown="True" w223 {
                tunnel: [w244 w250] -> w220
                tunnel: w217 -> [w243 w249]
                tunnel: [w243 w248] -> w216
                tunnel: T5 {"Com Port"=1, "ISOBUS Address"=0, "GPIB Address"=25, "Communication"=enum."GPIB"} ("Address") -> [_ w247]
                frame False {
                  n101 = local read "Actual Temperature (K)"() -> (w244:dbl)
                }
                frame True {
                  # "Temperature/Magnet read"
                  n102 = local read "Magnet ON?"() -> (w245:bool)
                  n103 = local read "Lake Shore"() -> (w246:refnum<visa-resource-name>)
                  n104 = case shown="True" w245 {
                    tunnel: w247 -> [_ w257]
                    frame False {
                    }
                    frame True {
                      n105 = call "GPIB - BusCommand.vi"("Command"="R7" ("format string"), "Address"=w257) -> ("Reply"=w258:string)  [unwired: 1 out]
                      n106 = Scan From String(format string="R%f" ("remaining string"), input string=w258) -> (output 1=w256:dbl)  [unwired: 3 in, 3 out]
                      n107 = local write "Actual Field (T)"(w256) -> ()
                    }
                  }
                  n108 = VISA Write(VISA resource name=w246, write buffer="KRDG?a", error in (no error)=w249) -> (VISA resource name out=w254:refnum<visa-resource-name>, error out=w253:errorcluster)  [unwired: 1 out]
                  n109 = VISA Read(VISA resource name=w254, byte count=u32 1000, error in (no error)=w253) -> (read buffer=w251:string, error out=w248:errorcluster)  [unwired: 2 out]
                  n110 = Fract/Exp String To Number(string=w251) -> (number=w250:dbl)  [unwired: 3 in, 1 out]
                }
              }
              "Actual Temperature (K)" <- w220
              n111 = Build Array (concatenate)(w222, w220) -> (w221:dbl[])
              "Temperature array" <- w221
              n112 = case shown="True" "Sweep Field" {
                tunnel: [Mode."Plot" ("Enum") Mode."Sweep" ("Enum")] -> w219
                frame False {
                }
                frame True {
                }
              }
            }
            frame "Sweep" {
              n113 = local read "Actual Field (T)"() -> (w285:dbl)
              n114 = local read "Min Field (T)"() -> (w284:dbl)
              n115 = local read "Max Field (T)"() -> (w283:dbl)
              n116 = local read "Read?"() -> (w288:bool)
              n117 = Equal?(x=w285, y=w284) -> (x = y?=w286:bool)
              n118 = And(x=w286, y=w288) -> (x .and. y?=w287:bool)
              n119 = case shown="True" w287 {
                tunnel: [w292 w323] -> w281
                tunnel: w283 -> [w290 w322]
                tunnel: w284 -> [_ w321]
                tunnel: w285 -> [_ w319]
                tunnel: w282 -> [w293 w318]
                frame True {
                  # "Ramp Up"
                  n120 = case shown="False" "First?" {
                    tunnel: [TRUE ("Save") FALSE ("Save")] -> w296
                    tunnel: [w310 w314] -> w295
                    frame False {
                      n121 = local read "Counter"() -> (w313:i8)
                      n122 = local write "Actual Polarization"(0.0 ("Actual Polarization")) -> ()
                      n123 = Increment(x=w313) -> (x+1=w310:i8)
                      n124 = local write "Counter"(w310) -> ()
                    }
                    frame True {
                      n125 = local read "Counter"() -> (w314:i8)
                      n126 = local write "First?"(FALSE ("First?")) -> ()
                    }
                  }
                  "Reset" <- w296
                  n127 = local write "Read?"(FALSE ("Read?")) -> ()
                  n128 = local read "Record ALL"() -> (w291:bool)
                  n129 = case shown="True" w291 {
                    tunnel: w295 -> [_ w303]
                    tunnel: [FALSE w301] -> w294
                    frame False {
                    }
                    frame True {
                      n130 = Greater?(x=w303, y="Max Countl") -> (0:w301:bool)
                    }
                  }
                  n131 = case shown="True" w294 {
                    tunnel: w293 -> [w306 w309]
                    tunnel: [w305 w309] -> w292
                    tunnel: w290 -> [w304 _]
                    frame False {
                      n132 = call "Set_B.vi"("error in (no error)"=w306, "address string"="25", "Set Field (T)"=w304) -> ("error out"=w305:errorcluster)  [unwired: 8 in]
                    }
                    frame True {
                      "New" <- TRUE
                    }
                  }
                  n133 = Wait (ms)(milliseconds to wait=u32 1000) -> ()  [unwired: 1 out]
                  "Up/Down" <- FALSE ("Up/Down")
                }
                frame False {
                  n134 = Equal?(x=w322, y=w319) -> (x = y?=w320:bool)
                  n135 = case shown="True" w320 {
                    tunnel: [w324 w328] -> w323
                    tunnel: w321 -> [_ _]
                    tunnel: w318 -> [w324 w329]
                    frame False {
                    }
                    frame True {
                      # "Resetting at the end of every cycle"
                      # "Ramp Dn"
                      n136 = local write "Up/Down"(TRUE ("Up/Down")) -> ()
                      n137 = local read "Min Field (T)"() -> (w327:dbl)
                      n138 = call "Set_B.vi"("error in (no error)"=w329, "address string"="25", "Set Field (T)"=w327) -> ("error out"=w328:errorcluster)  [unwired: 8 in]
                      n139 = local write "Reset"(TRUE ("Reset")) -> ()
                      n140 = Wait (ms)(milliseconds to wait=u32 1000) -> ()  [unwired: 1 out]
                    }
                  }
                  n141 = local write "Read?"(FALSE ("Read?")) -> ()
                }
              }
            }
            frame "Plot" {
              # "dI"
              n142 = local read "P(uC/mm^2)"() -> (w333:dbl[])
              n143 = local read "Actual Polarization"() -> (w332:dbl)
              n144 = local read "Actual Current (pA)"() -> (w334:dbl)
              n145 = local read "Time Lag"() -> (w346:dbl)
              n146 = Multiply(x=w334, y=w346) -> (x*y=w338:dbl)
              n147 = Divide(x=w338, y="Sample area (mm^2)") -> (x/y=w337:dbl)
              n148 = Add(x=w337, y=w332) -> (x+y=w336:dbl)
              "Actual Polarization" <- w336
              n149 = local read "Temp/Magnetic Field"() -> (w347:bool)
              n150 = Build Array (concatenate)(w333, w336) -> (→"P(uC/mm^2)":dbl[])
              n151 = case shown="True" w347 {
                tunnel: w344 -> [_ w407]
                tunnel: w341 -> [_ w389]
                tunnel: w336 -> [w354 w390]
                frame False {
                  # "Magnetic Field plotting"
                  n152 = local read "Up/Down"() -> (w359:bool)
                  n153 = local read "Actual B Field (T)"() -> (w356:dbl)
                  n154 = case shown="False" w359 {
                    frame True {
                      # "Down"
                      n155 = local read "I(B) 3"() -> (w369:cluster{dbl[], dbl[]}[])
                      n156 = local read "I(B) 3"() -> (w373:cluster{dbl[], dbl[]}[])
                      n157 = Index Array(array=w369, index=1) -> (element=w367:cluster{dbl[], dbl[]})
                      n158 = Unbundle(w367) -> (w366:dbl[], w365:dbl[])
                      n159 = Index Array(array=w373, index=i8 0 ("t")) -> (element=w370:cluster{dbl[], dbl[]})
                      n160 = local read "Actual Current (pA)"() -> (w362:dbl)
                      n161 = local read "Actual B Field (T)"() -> (w361:dbl)
                      n162 = Build Array (concatenate)(w366, w361) -> (w364:dbl[])
                      n163 = Build Array (concatenate)(w365, w362) -> (w363:dbl[])
                      n164 = Bundle(w364, w363) -> (w360:cluster{dbl[], dbl[]})  [unwired: 1 in]
                      n165 = Build Array(w370, w360) -> (w371:cluster{dbl[], dbl[]}[])
                      n166 = local write "I(B) 3"(w371) -> ()
                    }
                    frame False {
                      # "Up"
                      n167 = local read "I(B) 3"() -> (w385:cluster{dbl[], dbl[]}[])
                      n168 = local read "I(B) 3"() -> (w387:cluster{dbl[], dbl[]}[])
                      n169 = Index Array(array=w385, index=0) -> (element=w383:cluster{dbl[], dbl[]})
                      n170 = Unbundle(w383) -> (w382:dbl[], w381:dbl[])
                      n171 = Index Array(array=w387, index=i8 1 ("t")) -> (element=w375:cluster{dbl[], dbl[]})
                      n172 = local read "Actual B Field (T)"() -> (w377:dbl)
                      n173 = local read "Actual Current (pA)"() -> (w376:dbl)
                      n174 = Build Array (concatenate)(w382, w377) -> (w380:dbl[])
                      n175 = Build Array (concatenate)(w381, w376) -> (w379:dbl[])
                      n176 = Bundle(w380, w379) -> (w378:cluster{dbl[], dbl[]})  [unwired: 1 in]
                      n177 = Build Array(w378, w375) -> (w374:cluster{dbl[], dbl[]}[])
                      n178 = local write "I(B) 3"(w374) -> ()
                    }
                  }
                  n179 = local read "P(B)"() -> (w358:cluster{"yi":dbl[], dbl[]})
                  n180 = Unbundle(w358) -> ("yi"=w357:dbl[], w355:dbl[])
                  n181 = Build Array (concatenate)(w357, w356) -> (w353:dbl[])
                  n182 = Build Array (concatenate)(w355, w354) -> (w352:dbl[])
                  n183 = Bundle(w353, w352) -> (→"P(B)":cluster{dbl[], dbl[]})  [unwired: 1 in]
                }
                frame True {
                  # "Temperature plotting"
                  n184 = Quotient & Remainder(x=w407, y="Save Period") -> (x-y*floor(x/y)=w388:dbl)  [unwired: 1 out]
                  n185 = Greater?(x=w389, y=w388) -> (0:w405:bool)
                  n186 = local read "Actual Temperature (K)"() -> (w392:dbl)
                  n187 = local read "Actual Current (pA)"() -> (w398:dbl)
                  n188 = local read "P(T)"() -> (w394:cluster{"yi":dbl[], dbl[]})
                  n189 = local read "I(T)"() -> (w404:cluster{dbl[], dbl[]})
                  n190 = case shown="True" w405 {
                    frame False {
                    }
                    frame True {
                      n191 = local write "Reset"(TRUE) -> ()
                    }
                  }
                  n192 = Unbundle(w394) -> ("yi"=w395:dbl[], w391:dbl[])
                  n193 = Unbundle(w404) -> (w402:dbl[], w401:dbl[])
                  n194 = Build Array (concatenate)(w395, w392) -> (w396:dbl[])
                  n195 = Build Array (concatenate)(w391, w390) -> (w397:dbl[])
                  n196 = Build Array (concatenate)(w402, w392) -> (w400:dbl[])
                  n197 = Build Array (concatenate)(w401, w398) -> (w399:dbl[])
                  n198 = Bundle(w400, w399) -> (→"I(T)":cluster{dbl[], dbl[]})  [unwired: 1 in]
                  n199 = Bundle(w396, w397) -> (→"P(T)":cluster{dbl[], dbl[]})  [unwired: 1 in]
                }
              }
            }
            frame "Save" {
              n200 = local read "Reset"() -> (w409:bool)
              n201 = case shown="True" w409 {
                tunnel: w414 -> [w431 w433]
                tunnel: [w431 w436] -> w419
                tunnel: w413 -> [w430 w434]
                tunnel: [w430 w436] -> w418
                tunnel: w415 -> [w429 w435]
                tunnel: [w429 w436] -> w417
                tunnel: [w428 w436] -> w416
                tunnel: w412 -> [w428 w432]
                frame False {
                }
                frame True {
                  n202 = stacked-sequence {
                    tunnel: [_ _ w473] -> w436
                    tunnel: w435 -> [_ w462 _]
                    tunnel: w434 -> [w447 w460 _]
                    tunnel: w433 -> [w448 w461 _]
                    tunnel: w432 -> [_ w458 _]
                    frame #0 {
                      n203 = local read "B array"() -> (w438:dbl[])
                      n204 = local read "Counter"() -> (w446:i8)
                      n205 = local read "Averaged I(B)"() -> (w450:dbl[][])
                      n206 = local read "Up/Down"() -> (w449:bool)
                      n207 = call "Average_IB_curves.vi"("B array"=w438, "Up/Down"=w449, "Counter"=w446, "B in"=w448, "Averaged I(B) In"=w450, "I in"=w447) -> ("Averaged I(B) out"=w441:dbl[][])  [unwired: 5 in]
                      "Averaged I(B)" <- w441
                      n208 = Index Array(array=w441, index (row)=0 ("disabled index (col)")) -> (element=w439:dbl[])  [unwired: 1 in]
                      n209 = Index Array(array=w441, index (row)=1 ("disabled index (col)")) -> (element=w437:dbl[])  [unwired: 1 in]
                      n210 = Bundle("B array"=w438, "Averaged I(B) out"=w439) -> (w445:T7)  [unwired: 1 in]
                      n211 = Bundle("B array"=w438, "Averaged I(B) out"=w437) -> (w444:T7)  [unwired: 1 in]
                      n212 = Build Array(w445, w444) -> (→"I(B) /Averaged/ 2":T8)
                    }
                    frame #1 {
                      # "Save and Reset"
                      n213 = local read "Temp/Magnetic Field"() -> (w451:bool)
                      n214 = local read "Measurement File"() -> (w453:path)
                      n215 = local read "P(uC/mm^2)"() -> (w459:dbl[])
                      n216 = Build Array(w462, w461, w460, w458, w459) -> (w452:dbl[][])
                      n217 = case shown="False" w451 {
                        tunnel: w453 -> [_ _]
                        tunnel: w452 -> [w467 _]
                        frame False {
                          n218 = local read "Up/Down"() -> (w465:bool)
                          n219 = case shown="False" w465 {
                            tunnel: [w470 w471] -> w464
                            frame False {
                              n220 = local read "Measurement File_dn"() -> (w470:path)
                            }
                            frame True {
                              n221 = local read "Measurement File_up"() -> (w471:path)
                            }
                          }
                          n222 = call-poly <vilib>:"Write Delimited Spreadsheet.vi"("file path (dialog if empty)"=w464, "format (%.3f)"="%.5g", "2D data"=w467, "append to file? (F)"=TRUE ("transpose? (F)"), "transpose? (F)"=FALSE ("append to file? (F)")) -> ()  [unwired: 9 in, 2 out]
                        }
                        frame True {
                        }
                      }
                      n223 = case shown="False" "Reset IB?" {
                        frame False {
                        }
                        frame True {
                          n224 = local read "Up/Down"() -> (w472:bool)
                          n225 = case shown="False" w472 {
                            frame False {
                              n226 = invoke on="I(B) 3" class="XYGraph (strict)" method="Reinit To Default"() -> ()  [unwired: 3 in, 3 out]
                            }
                            frame True {
                            }
                          }
                        }
                      }
                      n227 = call-poly <vilib>:"Write Delimited Spreadsheet.vi"("file path (dialog if empty)"=w453, "format (%.3f)"="%.5g", "2D data"=w452, "append to file? (F)"=TRUE, "transpose? (F)"=TRUE) -> ()  [unwired: 9 in, 2 out]
                      n228 = local write "Reset"(FALSE ("Save")) -> ()
                    }
                    frame #2 {
                      w473 = dbl[] []
                      n229 = local write "P(uC/mm^2)"(w473) -> ()
                    }
                  }
                }
              }
              n230 = local read "New"() -> (w411:bool)
              n231 = case shown="True" w411 {
                tunnel: [Mode."Return" ("Enum") Mode."New" ("Enum")] -> w423
                tunnel: [TRUE FALSE] -> w410
                frame False {
                }
                frame True {
                }
              }
            }
            frame "New" {
              n232 = stacked-sequence {
                seq-local: [_ _ _ _ w564 _ _] -> [_ _ _ _ _ w573 _]
                seq-local: [_ _ w521 _ _ _ _] -> [_ _ _ _ w563 _ _]
                tunnel: T5 {"Com Port"=1, "ISOBUS Address"=0, "GPIB Address"=25, "Communication"=enum."GPIB"} ("Address") -> [_ _ w520 w558 _ _ _]
                tunnel: w476 -> [_ _ w522 _ _ w574 _]
                tunnel: [_ _ _ _ _ w576 _] -> w475
                tunnel: w474 -> [_ w501 _ _ _ _ _]
                frame #0 {
                  # "Save averages"
                  n233 = local read "Measurement File_average"() -> (w489:path)
                  n234 = local read "I(B) /Averaged/ 2"() -> (w490:cluster{"B array":dbl[], dbl[]}[])
                  n235 = Index Array(array=w490, index=0) -> (element=w493:cluster{"B array":dbl[], dbl[]})
                  n236 = Index Array(array=w490, index=1) -> (element=w494:cluster{"B array":dbl[], dbl[]})
                  n237 = Unbundle(w493) -> ("B array"=w495:dbl[], w496:dbl[])
                  n238 = Unbundle(w494) -> ("B array"=w497:dbl[], w498:dbl[])
                  n239 = Build Array(w495, w496, w497, w498) -> (w499:dbl[][])
                  n240 = call-poly <vilib>:"Write Delimited Spreadsheet.vi"("file path (dialog if empty)"=w489, "format (%.3f)"="%.5g", "2D data"=w499, "append to file? (F)"=TRUE ("transpose? (F)"), "transpose? (F)"=TRUE ("append to file? (F)")) -> ()  [unwired: 9 in, 2 out]
                }
                frame #1 {
                  w507 = dbl[] []
                  w516 = dbl[] []
                  # "Reset Flags"
                  n241 = Get Date/Time In Seconds() -> (seconds since 1Jan1904=w517:timestamp)
                  n242 = local write "Up/Down"(TRUE ("Up/Down")) -> ()
                  n243 = local write "First?"(TRUE ("First?")) -> ()
                  n244 = local write "Offset?"(FALSE ("Offset?")) -> ()
                  n245 = local write "New"(FALSE ("New")) -> ()
                  n246 = local write "P(uC/mm^2)"(w516) -> ()
                  n247 = local write "Start time"(w517) -> ()
                  n248 = local write "Offset array"(w516) -> ()
                  n249 = local write "Actual Polarization"(0.0 ("Actual Polarization")) -> ()
                  n250 = local write "Up/Down"(TRUE ("Up/Down")) -> ()
                  n251 = local write "Reset"(FALSE ("Reset")) -> ()
                  n252 = local read "B array"() -> (w510:dbl[])
                  n253 = local write "Counter"(i8 0 ("Counter")) -> ()
                  n254 = invoke on="P(B)" class="XYGraph (strict)" method="Reinit To Default"() -> ()  [unwired: 3 in, 3 out]
                  n255 = invoke on="I(B) 3" class="XYGraph (strict)" method="Reinit To Default"() -> ()  [unwired: 3 in, 3 out]
                  n256 = Multiply(x=w510, y=0.0) -> (x*y=w511:dbl[])
                  n257 = Build Array(w507, w507) -> (w515:dbl[][])
                  n258 = Bundle("B array"=w510, w511) -> (w512:cluster{"B array":dbl[], dbl[]})  [unwired: 1 in]
                  n259 = local write "Averaged I(B)"(w515) -> ()
                  n260 = Build Array(w512, w512) -> (w513:cluster{"B array":dbl[], dbl[]}[])
                  n261 = local write "I(B) /Averaged/ 2"(w513) -> ()
                  n262 = local write "Measuring"(FALSE ("Measuring")) -> ()
                  n263 = Flush Queue(queue=w501) -> (remaining elements=→"remaining elements":T1)  [unwired: 1 in, 2 out]
                }
                frame #2 {
                  # "Step"
                  n264 = local read "Sweep Rate Array"() -> (w526:dbl[])
                  n265 = local read "j"() -> (w527:i32)
                  n266 = Increment(x=w527) -> (x+1=w523:i32)
                  n267 = Array Size(array=w526) -> (size(s)=w525:i32)
                  n268 = Less?(x=w523, y=w525) -> (x < y?=w524:bool)
                  "Step Rate" <- w524
                  n269 = case shown="False" w524 {
                    tunnel: w523 -> [_ w554]
                    tunnel: w522 -> [w530 w553]
                    tunnel: [w529 w553] -> w521
                    tunnel: w520 -> [w528 _]
                    frame False {
                      # "Step Temp?"
                      n270 = local read "Temperature Array"() -> (w534:dbl[])
                      n271 = local read "i"() -> (w535:i32)
                      n272 = Increment(x=w535) -> (x+1=w532:i32)
                      n273 = local write "j"(0 ("f")) -> ()
                      n274 = Array Size(array=w534) -> (size(s)=w533:i32)
                      n275 = Less?(x=w532, y=w533) -> (x < y?=w531:bool)
                      "Step Temp" <- w531
                      n276 = case shown="False" w531 {
                        tunnel: w532 -> [_ w552]
                        tunnel: w530 -> [w540 w551]
                        tunnel: [w539 w551] -> w529
                        tunnel: w528 -> [w538 _]
                        frame False {
                          # "Heater OFF"
                          # "Finished"
                          n277 = local write "i"(0 ("i")) -> ()
                          n278 = stacked-sequence {
                            tunnel: w540 -> [w544 _ _]
                            tunnel: [w543 _ _] -> w539
                            tunnel: w538 -> [_ w548 w549]
                            frame #0 {
                              n279 = local read "Lake Shore"() -> (w545:refnum<visa-resource-name>)
                              n280 = VISA Write(VISA resource name=w545, write buffer="RANGE,1,0", error in (no error)=w544) -> (error out=w543:errorcluster)  [unwired: 2 out]
                            }
                            frame #1 {
                              n281 = call "ips_switchHeaterOff.vi"("Instrument address"=w548, "Rate"=2.0) -> ()  [unwired: 1 out]
                            }
                            frame #2 {
                              n282 = call "GPIB - BusCommand.vi"("Command"="H0", "Address"=w549) -> ()  [unwired: 2 out]
                            }
                          }
                          n283 = local write "Record ALL"(FALSE ("Record ALL")) -> ()
                          "Finished" <- TRUE
                        }
                        frame True {
                          n284 = local write "i"(w552) -> ()
                        }
                      }
                    }
                    frame True {
                      n285 = local write "j"(w554) -> ()
                    }
                  }
                }
                frame #3 {
                  # "Set rates"
                  n286 = local read "Sweep Rate Array"() -> (w557:dbl[])
                  n287 = local read "j"() -> (w556:i32)
                  n288 = Index Array(array=w557, index=w556) -> (element=w555:dbl)
                  n289 = Number To Fractional String(number=w555, precision (6)=i16 3) -> (F-format string=w561:string)  [unwired: 2 in]
                  n290 = Concatenate Strings("T" ("format string"), w561) -> (w562:string)
                  n291 = call "GPIB - BusCommand.vi"("Command"=w562, "Address"=w558) -> ()  [unwired: 2 out]
                  n292 = local write "Sweep Rate (T/min)"(w555) -> ()
                }
                frame #4 {
                  # "Set temperature"
                  n293 = local read "Temperature Array"() -> (w567:dbl[])
                  n294 = local read "i"() -> (w566:i32)
                  n295 = Index Array(array=w567, index=w566) -> (element=w565:dbl)
                  n296 = local read "Lake Shore"() -> (w569:refnum<visa-resource-name>)
                  n297 = Number To Fractional String(number=w565, precision (6)=i16 3) -> (F-format string=w570:string)  [unwired: 2 in]
                  n298 = Concatenate Strings("SETP 1," ("write buffer"), w570) -> (w572:string)
                  n299 = VISA Write(VISA resource name=w569, write buffer=w572, error in (no error)=w563) -> (error out=w564:errorcluster)  [unwired: 2 out]
                }
                frame #5 {
                  n300 = local read "Finished"() -> (w575:bool)
                  n301 = case shown="False" w575 {
                    tunnel: [w582 w621] -> w576
                    tunnel: w574 -> [_ _]
                    tunnel: w573 -> [w579 w621]
                    frame False {
                      w577 = "_" ("string")
                      # "Wait, create Files"
                      n302 = local read "Temperature Array"() -> (w611:dbl[])
                      n303 = local read "Sweep Rate Array"() -> (w607:dbl[])
                      n304 = local read "i"() -> (w610:i32)
                      n305 = local read "j"() -> (w608:i32)
                      n306 = Index Array(array=w611, index=w610) -> (element=w609:dbl)
                      n307 = Index Array(array=w607, index=w608) -> (element=w606:dbl)
                      n308 = Number To Fractional String(use system decimal point (T)=TRUE, number=w606, precision (6)=i16 1) -> (F-format string=w578:string)  [unwired: 1 in]
                      n309 = Number To Fractional String(use system decimal point (T)=TRUE, number=w609, precision (6)=i16 1) -> (F-format string=w612:string)  [unwired: 1 in]
                      n310 = Concatenate Strings("Directory", "\\" ("string"), "FileName", w577, w612, "K" ("string"), w577, w578, "Tpm" ("string")) -> (w599:string)
                      n311 = Search and Replace String(replace all?=TRUE ("replace all? (F)"), input string=w599, search string=".", replace string="p" ("substring (\"\")"), error in=w579) -> (result string=w594:string, error out=w589:errorcluster)  [unwired: 3 in, 2 out]
                      n312 = local write "Step Rate"(FALSE ("Step Rate")) -> ()
                      n313 = Concatenate Strings(w594, ".txt" ("string")) -> (w593:string)
                      n314 = local read "Step Temp"() -> (w583:bool)
                      n315 = String To Path(string=w593) -> (path=w592:path)
                      n316 = Open/Create/Replace File(file path (use dialog)=w592, error in=w589, operation (0:open)=T4."open or create") -> (refnum out=w581:refnum<file>, error out=w582:errorcluster)  [unwired: 3 in, 1 out]
                      n317 = local write "refnum out"(w581) -> ()
                      n318 = Refnum to Path(1:w581) -> (0:w584:path)
                      n319 = call "Create_sweep_files.vi"("Measurement File"=w584) -> ("Path 3"=w587:path, "Path 2"=w586:path, "Path"=w585:path)  [unwired: 8 in]
                      n320 = local write "Measurement File"(w584) -> ()
                      n321 = case shown="True" w583 {
                        frame False {
                        }
                        frame True {
                          n322 = Get Date/Time In Seconds() -> (seconds since 1Jan1904=w614:timestamp)
                          n323 = local write "Step Temp"(FALSE ("Step Temp")) -> ()
                          n324 = while {
                            tunnel: w614 -> [w619]
                            stop <- w616 stop-if-true
                            n325 = Get Date/Time In Seconds() -> (seconds since 1Jan1904=w620:timestamp)
                            n326 = Subtract(x=w620, y=w619) -> (x-y=w618:dbl)
                            "Wait (s)" <- w618
                            n327 = Greater Or Equal?(x=w618, y="secs to wait") -> (x >= y?=w616:bool)
                          }
                        }
                      }
                      n328 = local write "Measurement File_dn"(w587) -> ()
                      n329 = local write "Measurement File_average"(w585) -> ()
                      n330 = local write "Measurement File_up"(w586) -> ()
                    }
                    frame True {
                    }
                  }
                }
                frame #6 {
                  n331 = local read "Finished"() -> (w622:bool)
                  n332 = case shown="True" w622 {
                    frame False {
                      n333 = local write "Measuring"(TRUE ("Measuring")) -> ()
                    }
                    frame True {
                      n334 = local write "Measure /Pause"(FALSE ("Measure /Pause")) -> ()
                    }
                  }
                }
              }
            }
            frame "Return" {
            }
          }
        }
      }
      frame Error {
        # "Return true for any case which should stop the loop."
      }
    }
  }
  n335 = case shown="True" w2 {
    frame False {
    }
    frame True {
      n336 = invoke on="P(T)" class="XYGraph (strict)" method="Reinit To Default"() -> ()  [unwired: 3 in, 3 out]
      n337 = invoke on="I(T)" class="XYGraph (strict)" method="Reinit To Default"() -> ()  [unwired: 3 in, 3 out]
    }
  }
  n338 = while {
    shift-right: [w653] -> w49
    shift-left: w26 -> [w654]
    shift-right: [w655] -> w56
    shift-left: w57 -> [w656]
    tunnel: w52 -> [w652]
    tunnel: w51 -> [w651]
    tunnel: w29 -> [w650]
    tunnel: [w644] -> _
    tunnel: w36 -> [w643]
    tunnel: w24 -> [w642]
    stop <- "stop" stop-if-true
    n339 = event shown="[6] \"Stop\": Value Change" {
      selector: _ -> [_ _ _ _ _ _ _ _ _ _ _ _ _ _ _]
      dyn-events: _ -> [_ _ _ _ _ _ _ _ _ _ _ _ _ _ _]
      timeout: 10 -> [_ _ _ _ _ _ _ _ _ _ _ _ _ _ _]
      tunnel: w656 -> [w666 w698 w707 w715 w726 w731 w735 w761 w777 w794 w837 w854 w870 w880 w891]
      tunnel: [w665 w698 w707 w715 w726 w731 w735 w761 w777 w794 w837 w854 w870 w880 w891] -> w655
      tunnel: w654 -> [w664 w697 w706 w716 w725 w733 w737 w762 w776 w793 w838 w856 w874 w884 w893]
      tunnel: [w663 w697 w706 w716 w727 w733 w736 _ w776 w793 w838 w855 w873 w883 w892] -> w653
      tunnel: w652 -> [w662 _ _ _ _ _ _ _ _ _ _ _ _ _ _]
      tunnel: w651 -> [w661 _ _ _ _ _ _ _ _ _ _ _ _ _ _]
      tunnel: w650 -> [w660 _ _ _ _ _ _ _ _ _ _ _ _ _ _]
      tunnel: [w658 w696 w705 w714 w728 w732 w734 w760 w775 w792 w836 w853 w871 w881 _] -> w644
      tunnel: w643 -> [w658 w696 w708 w714 w728 w732 w734 w760 w775 w792 w836 w853 w871 w881 _]
      tunnel: w642 -> [_ _ _ _ _ _ _ _ _ _ _ w857 w872 w885 w890]
      tunnel: [_ _ _ _ _ _ _ w762 _ _ _ _ _ _ _] -> _
      event Timeout {
        n340 = event-data() -> ()  [unwired: 1 in, 3 out]
        n341 = case shown="True" "Measuring" {
          tunnel: w666 -> [w668 w687]
          tunnel: [w668 w686] -> w665
          tunnel: w664 -> [w667 _]
          tunnel: [w667 w685] -> w663
          tunnel: w662 -> [_ w678]
          tunnel: w661 -> [_ w677]
          tunnel: w660 -> [_ w672]
          frame False {
          }
          frame True {
            w675 = ":FETCh? " ("data")
            w679 = u32 1000 ("byte count")
            # "Generate the data here."
            n342 = case shown="No Error" w672 {
              selector: w672 -> [w689 w690]
              tunnel: [w689 w690] -> w671
              tunnel: [w688 _] -> w670
              frame No Error {
                n343 = Get Date/Time In Seconds() -> (seconds since 1Jan1904=w688:timestamp)
              }
              frame Error {
              }
            }
            n344 = VISA Write(VISA resource name=w678, write buffer=w675, error in (no error)=w671) -> (VISA resource name out=w684:refnum<visa-resource-name>, error out=w682:errorcluster)  [unwired: 1 out]
            n345 = VISA Write(VISA resource name=w677, write buffer=w675, error in (no error)=w682) -> (VISA resource name out=w683:refnum<visa-resource-name>, error out=w681:errorcluster)  [unwired: 1 out]
            n346 = VISA Read(VISA resource name=w684, byte count=w679, error in (no error)=w681) -> (read buffer=w673:string, error out=w680:errorcluster)  [unwired: 2 out]
            n347 = VISA Read(VISA resource name=w683, byte count=w679, error in (no error)=w680) -> (read buffer=w674:string, error out=w676:errorcluster)  [unwired: 2 out]
            n348 = Bundle("seconds since 1Jan1904"=w670, "read buffer"=w673, "read buffer"=w674) -> (w669:T6)  [unwired: 1 in]
            n349 = Enqueue Element(queue=w687, element=w669, error in (no error)=w676) -> (queue out=w686:refnum<queue>, error out=w685:errorcluster)  [unwired: 1 in, 1 out]
          }
        }
      }
      event "Max Field (T)": Value Change {
        n350 = event-data() -> ()  [unwired: 1 in, 6 out]
        n351 = Divide(x="Max Field (T)", y="dB (T)") -> (x/y=w693:dbl)
        n352 = for {
          N: w693 -> [_]
          tunnel: "dB (T)" -> [w703]
          tunnel: [w700] -> w692 mode=indexing
          tunnel: "Min Field (T)" -> [w701]
          tunnel: [0.0] -> _ mode=indexing
          i -> [w704]
          n353 = Multiply(x=w704, y=w703) -> (x*y=w702:dbl)
          n354 = Add(x=w702, y=w701) -> (x+y=w700:dbl)
        }
        "B array" <- w692
      }
      event "Sweep Rate (T/min)": Value Change {
        n355 = event-data() -> ("NewVal"=w712:dbl)  [unwired: 1 in, 5 out]
        n356 = Number To Fractional String(number=w712, precision (6)=i16 3) -> (F-format string=w710:string)  [unwired: 2 in]
        n357 = Concatenate Strings("T" ("format string"), w710) -> (w709:string)
        n358 = call "GPIB - BusCommand.vi"("Command"=w709, "Address"=w708) -> ("Address(thru)"=w705:T5)  [unwired: 1 out]
      }
      event "Field To Zero": Value Change {
        n359 = event-data() -> ()  [unwired: 1 in, 6 out]
        n360 = Two Button Dialog(message="Do you want to switch off the field?", 1:"No" ("F button name (\"Cancel\")"), 2:"Yes" ("T button name (\"OK\")")) -> (T button?=w720:bool)
        n361 = case shown="True" w720 {
          tunnel: w714 -> [_ w723]
          frame False {
          }
          frame True {
            n362 = local read "Sweep Rate (T/min)"() -> (w722:dbl)
            n363 = call "ips_switchHeaterOff.vi"("Instrument address"=w723, "Rate"=w722) -> ("B"=w721:dbl)
            n364 = local write "Actual Field (T)"(w721) -> ()
          }
        }
      }
      event "Go to Set": Value Change {
        n365 = event-data() -> ()  [unwired: 1 in, 6 out]
        n366 = call "Set_B.vi"("error in (no error)"=w725, "address string"="25", "Set Field (T)"="Set Field (T)") -> ("error out"=w727:errorcluster)  [unwired: 8 in]
      }
      event "Measure /Pause": Value Change {
        n367 = event-data() -> ("NewVal"=w730:bool)  [unwired: 1 in, 5 out]
        n368 = local write "Measuring"(w730) -> ()
      }
      event "Stop": Value Change {
        n369 = event-data() -> ()  [unwired: 1 in, 6 out]
        n370 = local read "Measuring"() -> (w738:bool)
        n371 = case shown="True" w738 {
          tunnel: w737 -> [w739 w742]
          tunnel: [w739 w741] -> w736
          frame False {
          }
          frame True {
            w740 = FALSE ("Measuring")
            n372 = local read "SaveSweep"() -> (w745:bool)
            n373 = local write "Measuring"(w740) -> ()
            n374 = local read "Set Field (T)"() -> (w743:dbl)
            n375 = local write "Measure /Pause"(w740) -> ()
            n376 = case shown="True" w745 {
              frame False {
              }
              frame True {
                n377 = local read "Measurement File_average"() -> (w756:path)
                n378 = local read "I(B) /Averaged/ 2"() -> (w755:cluster{"B array":dbl[], dbl[]}[])
                n379 = Index Array(array=w755, index=0) -> (element=w752:cluster{"B array":dbl[], dbl[]})
                n380 = Index Array(array=w755, index=1) -> (element=w751:cluster{"B array":dbl[], dbl[]})
                n381 = Unbundle(w752) -> ("B array"=w750:dbl[], w749:dbl[])
                n382 = Unbundle(w751) -> ("B array"=w748:dbl[], w747:dbl[])
                n383 = Build Array(w750, w749, w748, w747) -> (w746:dbl[][])
                n384 = call-poly <vilib>:"Write Delimited Spreadsheet.vi"("file path (dialog if empty)"=w756, "format (%.3f)"="%.5g", "2D data"=w746, "append to file? (F)"=TRUE ("transpose? (F)"), "transpose? (F)"=TRUE ("append to file? (F)")) -> ()  [unwired: 9 in, 2 out]
              }
            }
            n385 = call "Set_B.vi"("error in (no error)"=w742, "address string"="25", "Set Field (T)"=w743) -> ("error out"=w741:errorcluster)  [unwired: 8 in]
          }
        }
      }
      event "Sweep Field": Value Change {
        n386 = event-data() -> ("NewVal"=w763:bool)  [unwired: 1 in, 5 out]
        n387 = case shown="True" w763 {
          frame False {
          }
          frame True {
            n388 = local read "Measurement File"() -> (w764:path)
            n389 = Two Button Dialog(message="Do you want to create additional files for the sweeping measurements?" ("string"), 1:"No" ("F button name (\"Cancel\")"), 2:"Yes" ("T button name (\"OK\")")) -> (T button?=w766:bool)
            n390 = case shown="True" w766 {
              tunnel: w764 -> [_ w771]
              frame False {
                n391 = local write "SaveSweep"(FALSE ("SaveSweep")) -> ()
              }
              frame True {
                n392 = call "Create_sweep_files.vi"("Measurement File"=w771) -> ("Path 3"=→"Measurement File_dn":path, "Path 2"=→"Measurement File_up":path, "Path"=→"Measurement File_average":path)  [unwired: 8 in]
                "SaveSweep" <- TRUE
              }
            }
          }
        }
      }
      event "Measure Noise": Value Change {
        n393 = event-data() -> ("NewVal"=w778:bool)  [unwired: 1 in, 5 out]
        n394 = case shown="True" w778 {
          frame False {
          }
          frame True {
            n395 = local read "Gain (V/A)"() -> (w783:dbl)
            n396 = call "Noise_measurement.vi"("Gain (V/A)"=w783, "Cycles"="Cycles", "Lower Cut-Off"="Cut-Off Frequency", "minimum value"="minimum value", "Filter On"="Filter On", "maximum value"="maximum value", "physical channels"="physical channels", "rate"="Rate", "samples per channel"="Samples per channel") -> ("Current (pA) Filtered"=→"Current (pA) Filtered":waveform(dbl), "PSD (pA/Hz^1/2) Peaks Removed"=→"PSD (pA/Hz^1/2) Peaks Removed":cluster{"f0":dbl, "df":dbl, "magnitude":dbl[]}, "Current (pA)"=→"Current (pA)":dbl[], "PSD (pA/Hz^1/2)"=→"PSD (pA/Hz^1/2)":cluster{"f0":dbl, "df":dbl, "magnitude":dbl[]})  [unwired: 3 in]
          }
        }
      }
      event "Calibrate": Value Change {
        n397 = event-data() -> ()  [unwired: 1 in, 6 out]
        n398 = case shown="True" "Calibrate" {
          frame False {
          }
          frame True {
            w798 = dbl[] []
            n399 = while {
              shift-right: [w831] -> w796
              shift-left: dbl[][] [] -> [w830]
              shift-right: [w814] -> _
              shift-left: w798 -> [w826]
              shift-right: [w823] -> _
              shift-left: w798 -> [w825]
              shift-right: [w813] -> _
              shift-left: w798 -> [w824]
              shift-right: [w805] -> _
              shift-left: 0.0 ("Set Field out") -> [w804]
              stop <- w827 stop-if-true
              n400 = call "Calibtarion.vi"("Dwell Time (ms)"="Dwell Time (ms)", "V array in (V)"=w826, "I array in (A)"=w824, "Collected array in"=w830, "B array in (T)"=w825, "Set Field (T)"=w804, "dB"="dB") -> ("Best Linear Fit"=w815:dbl[], "appended array"=→"appended array":dbl[][], "slope"=→"B/V (T/V)":dbl, "V array out (V)"=w814:dbl[], "Boolean"=w829:bool, "I array out (A)"=w813:dbl[], "intercept 2"=→"I0 (A)":dbl, "Collected array out"=w831:dbl[][], "intercept"=→"B0 (T)":dbl, "B array Out"=w823:dbl[], "slope 2"=→"V/I (Ohm)":dbl, "Best Linear Fit 2"=w820:dbl[], "Set Field out"=w805:dbl)
              n401 = Bundle("I array out (A)"=w813, "V array out (V)"=w814) -> (w822:T9)  [unwired: 1 in]
              n402 = Bundle("I array out (A)"=w813, "Best Linear Fit"=w815) -> (w816:T10)  [unwired: 1 in]
              n403 = Bundle("V array out (V)"=w814, "B array Out"=w823) -> (w818:T11)  [unwired: 1 in]
              n404 = Bundle("V array out (V)"=w814, "Best Linear Fit 2"=w820) -> (w819:T12)  [unwired: 1 in]
              n405 = Or(x=w829, y="stop 2") -> (x .or. y?=w827:bool)
              n406 = Build Array(w822, w816) -> (→"V_I":T13)
              n407 = Build Array(w818, w819) -> (→"B_V":T14)
            }
            n408 = flat-sequence {
              tunnel: w796 -> [w802]
              frame #0 {
                n409 = Two Button Dialog(message="Do you want to save calibration file?") -> (T button?=w801:bool)  [unwired: 2 in]
                n410 = case shown="True" w801 {
                  tunnel: w802 -> [_ w803]
                  frame False {
                  }
                  frame True {
                    n411 = call-poly <vilib>:"Write Delimited Spreadsheet.vi"("2D data"=w803) -> ()  [unwired: 13 in, 2 out]
                  }
                }
              }
            }
          }
        }
      }
      event "New Measurement File": Value Change {
        n412 = event-data() -> ()  [unwired: 1 in, 6 out]
        n413 = local read "Sweep Field"() -> (w833:bool)
        n414 = Open/Create/Replace File(prompt="Please select measurement file\n", operation (0:open)=T4."replace or create with confirmation") -> (refnum out=w839:refnum<file>)  [unwired: 4 in, 2 out]
        n415 = local write "refnum out"(w839) -> ()
        n416 = Refnum to Path(1:w839) -> (0:w834:path)
        n417 = case shown="True" w833 {
          tunnel: w834 -> [_ w842]
          frame False {
          }
          frame True {
            n418 = Two Button Dialog(message="Do you want to create additional files for the sweeping measurements?" ("string"), 1:"No" ("F button name (\"Cancel\")"), 2:"Yes" ("T button name (\"OK\")")) -> (T button?=w844:bool)
            n419 = case shown="False" w844 {
              tunnel: w842 -> [_ w852]
              frame False {
                n420 = local write "SaveSweep"(FALSE ("SaveSweep")) -> ()
              }
              frame True {
                n421 = call "Create_sweep_files.vi"("Measurement File"=w852) -> ("Path 3"=w849:path, "Path 2"=w850:path, "Path"=w851:path)  [unwired: 8 in]
                n422 = local write "Measurement File_dn"(w849) -> ()
                n423 = local write "Measurement File_average"(w851) -> ()
                n424 = local write "Measurement File_up"(w850) -> ()
                n425 = local write "SaveSweep"(TRUE) -> ()
              }
            }
          }
        }
        n426 = local write "Measurement File"(w834) -> ()
        n427 = local write "Offset?"(FALSE ("Offset?")) -> ()
        n428 = local write "First?"(TRUE ("First?")) -> ()
      }
      event "Heater On/Off": Value Change {
        n429 = event-data() -> ()  [unwired: 1 in, 6 out]
        n430 = case shown="False" "Heater On/Off" {
          tunnel: w857 -> [w862 w868]
          tunnel: w856 -> [w860 w869]
          tunnel: [w859 w867] -> w855
          frame False {
            n431 = VISA Write(VISA resource name=w862, write buffer="RANGE,1,0", error in (no error)=w860) -> (error out=w859:errorcluster)  [unwired: 2 out]
          }
          frame True {
            n432 = Number To Decimal String(number="Heater Range") -> (decimal integer string=w865:string)  [unwired: 1 in]
            n433 = Concatenate Strings("RANGE,1," ("write buffer"), w865) -> (w863:string)
            n434 = VISA Write(VISA resource name=w868, write buffer=w863, error in (no error)=w869) -> (error out=w867:errorcluster)  [unwired: 2 out]
          }
        }
      }
      event "Set temperature (K)": Value Change {
        n435 = event-data() -> ()  [unwired: 1 in, 6 out]
        n436 = local read "Set temperature (K)"() -> (w875:dbl)
        n437 = Number To Fractional String(number=w875, precision (6)=i16 3) -> (F-format string=w878:string)  [unwired: 2 in]
        n438 = Concatenate Strings("SETP 1," ("write buffer"), w878) -> (w876:string)
        n439 = VISA Write(VISA resource name=w872, write buffer=w876, error in (no error)=w874) -> (error out=w873:errorcluster)  [unwired: 2 out]
      }
      event "Temp Ramping Rate (K/min)": Value Change {
        n440 = event-data() -> ()  [unwired: 1 in, 6 out]
        n441 = local read "Temp Ramping Rate (K/min)"() -> (w882:dbl)
        n442 = Number To Fractional String(number=w882, precision (6)=i16 1) -> (F-format string=w888:string)  [unwired: 2 in]
        n443 = Concatenate Strings("RAMP 1,1," ("string"), w888) -> (w887:string)
        n444 = VISA Write(VISA resource name=w885, write buffer=w887, error in (no error)=w884) -> (error out=w883:errorcluster)  [unwired: 2 out]
      }
      event "Heater Range": Value Change {
        n445 = event-data() -> ()  [unwired: 1 in, 6 out]
        n446 = local read "Heater On/Off"() -> (w894:bool)
        n447 = case shown="True" w894 {
          tunnel: w893 -> [w895 w900]
          tunnel: [w895 w899] -> w892
          tunnel: w890 -> [_ w898]
          frame False {
          }
          frame True {
            n448 = local read "Heater Range"() -> (w896:enum16{"Off", "Low", "Medium", "High"})
            n449 = Number To Decimal String(number=w896) -> (decimal integer string=w902:string)  [unwired: 1 in]
            n450 = Concatenate Strings("RANGE,1," ("write buffer"), w902) -> (w901:string)
            n451 = VISA Write(VISA resource name=w898, write buffer=w901, error in (no error)=w900) -> (error out=w899:errorcluster)  [unwired: 2 out]
          }
        }
      }
    }
    n452 = Reciprocal(x="Sampling rate (Hz)") -> (1/x=w648:dbl)
    n453 = Multiply(x=w648, y=1000.0) -> (x*y=w646:dbl)
    n454 = Wait Until Next ms Multiple(millisecond multiple=w646) -> ()  [unwired: 1 out]
  }
  n455 = local read "Max Field (T)"() -> (w12:dbl)
  n456 = local read "Min Field (T)"() -> (w14:dbl)
  n457 = local read "dB (T)"() -> (w13:dbl)
  n458 = Divide(x=w12, y=w13) -> (x/y=w15:dbl)
  n459 = for {
    N: w15 -> [_]
    tunnel: w13 -> [w907]
    tunnel: [w904] -> w11 mode=indexing
    tunnel: w14 -> [w905]
    tunnel: [0.0] -> _ mode=indexing
    i -> [w908]
    n460 = Multiply(x=w908, y=w907) -> (x*y=w906:dbl)
    n461 = Add(x=w906, y=w905) -> (x+y=w904:dbl)
  }
  n462 = local write "B array"(w11) -> ()
  n463 = local read "Lake Shore"() -> (w27:refnum<visa-resource-name>)
  n464 = local read "IV converter"() -> (w47:refnum<visa-resource-name>)
  n465 = local read "Magnetic Field"() -> (w46:refnum<visa-resource-name>)
  n466 = VISA Close(VISA resource name=w47, error in (no error)=w49) -> (error out=w50:errorcluster)
  n467 = VISA Close(VISA resource name=w46, error in (no error)=w50) -> (error out=w48:errorcluster)
  n468 = Release Queue(queue=w56, error in (no error)=w48) -> (error out=w42:errorcluster)  [unwired: 1 in, 2 out]
  n469 = Merge Errors(w42, w41) -> (w43:errorcluster)
  n470 = VISA Close(VISA resource name=w27, error in (no error)=w43) -> (error out=w40:errorcluster)
  n471 = local read "refnum out"() -> (w38:refnum<file>)
  n472 = Close File(refnum=w38, error in=w40) -> (error out=w39:errorcluster)  [unwired: 1 out]
  n473 = call <vilib>:"Simple Error Handler.vi"("error in (no error)"=w39) -> ()  [unwired: 4 in, 5 out]
  "i" <- w3
  "j" <- w3
